vi "SubMatrixVgtmp.vi"(0 "Target Voltage, V":dbl=1.0 min=-4.0 max=4.0 step=0.1 format="%.4f", 2 "Sweep rate, V/min":dbl=0.1 min=0.0 max=1.0 step=0.01 format="%.4f", 3 "Custom Folder":string, 5 "optional Bias (V)":dbl=1e-08) -> ()   [LabVIEW 2014]
uses:
  <vilib>/Utility/file.llb/Write To Spreadsheet File (DBL).vi
panel:
  out "Comments":string[](array[string])
  out "ArrayBoolian":bool[][](array[boolean])
  out "Numeric 4":i32
  in  "Commutator":bool
  in  "Commute SorceMeter":enum32{"Radio Selection 1", "Radio Selection 2"}(radio)
  out "Numeric 3":i32
  in  "Channel 2 (Vnano3b)":bool
  in  "Channel 1 (Vnano3)":bool
  out "Numeric":i32
  in  "Capacitance (C) and Loss (L)":bool
  in  "Magnetic Field (B)":bool
  in  "Current (Ik3)":bool
  in  "Voltage (Vk3)":bool
  in  "Current (Ik2)":bool
  in  "Voltage (Vk2)":bool
  in  "Channel 2 (Vnano2b)":bool
  in  "Channel 1 (Vnano2)":bool
  in  "Thermometer 1 (T1)":bool=TRUE
  in  "Channel 2 (Vnano1b)":bool
  in  "Channel 1 (Vnano1)":bool
  in  "Current (Ik1)":bool=TRUE
  in  "Voltage (Vk1)":bool
  out "Numeric Current":dbl
  out "Main Keithly2614B address":string="12"
  out "Delib Time delay":i32
  in  "points at each Vg":i32=1
  out "XY Graph":cluster{dbl[], dbl[]}(graph)={[1.0, 0.8, 0.6000000000000001, 0.4000000000000001, 0.20000000000000007, 5.551115123125783e-17, -0.19999999999999996, -0.39999999999999997, -0.6, -0.8, -1.0], [0.03352775, 0.056811, 0.03911575, 0.04330675, -0.02468015, 0.011641600000000002, 0.10151450000000001, 0.12386675000000001, 0.08288825000000001, -0.00186266, -0.038650000000000004]}
  in  "Time btw \npoints, sec":dbl=1.0 format="%.2f"
  out "Array 2":dbl[][](array[numeric])
  out "array for data":dbl[](array[numeric])
  out "Array":string[](array[string])
  in  "Addr 1 lock-in oop":bool
  in  "Ring":u16(ring) caption="Y-axis:" items=["Vg", "I", "R1", "R1oop", "Ik1"]
  out "String":string
  out "Data file:":path
  in  "Set compliance limit, mkA":dbl=0.05 min=0.0 max=1.0 step=0.01 format="%.3f"
  in  "error in (no error)":errorcluster
  in  "Ring 3":u16(ring)=1 items=["1 kOhm", "10 kOhm", "100 kOhm", "1 Mohm", "10 mOhm"]
  in  "Ring 2":u16(ring)=3 items=["1 kOhm", "10 kOhm", "100 kOhm", "1 Mohm", "10 mOhm"]
  in  "Fixed Current mkA":dbl=1.0
  in  "Current is:":T1(radio)
  in  "Ressitance measurements?":bool=TRUE
  in  "Addr 5 lock-in oop":bool
  in  "Addr 4 lock-in oop":bool
  in  "Addr 3 lock-in oop":bool
  in  "Addr 2 lock-in oop":bool
  in  "Addr 5 lock-in":bool
  in  "Addr 4 lock-in":bool
  in  "Addr 3 lock-in":bool=TRUE
  in  "Addr 2 lock-in":bool=TRUE
  in  "Addr 1 lock-in":bool=TRUE
  # "Keithley 2400: address 12"
  # "0"
  # "SourceMeters"
  # "Nanovoltmeters"
  # "Temperature"
  # "Main"
  # "Magnetic Field"
  # "(not recommended, too slow)"
  # "Capacitance & Loss"
  # "(not recommended, too slow)"
  # "(not recommended, too slow)"
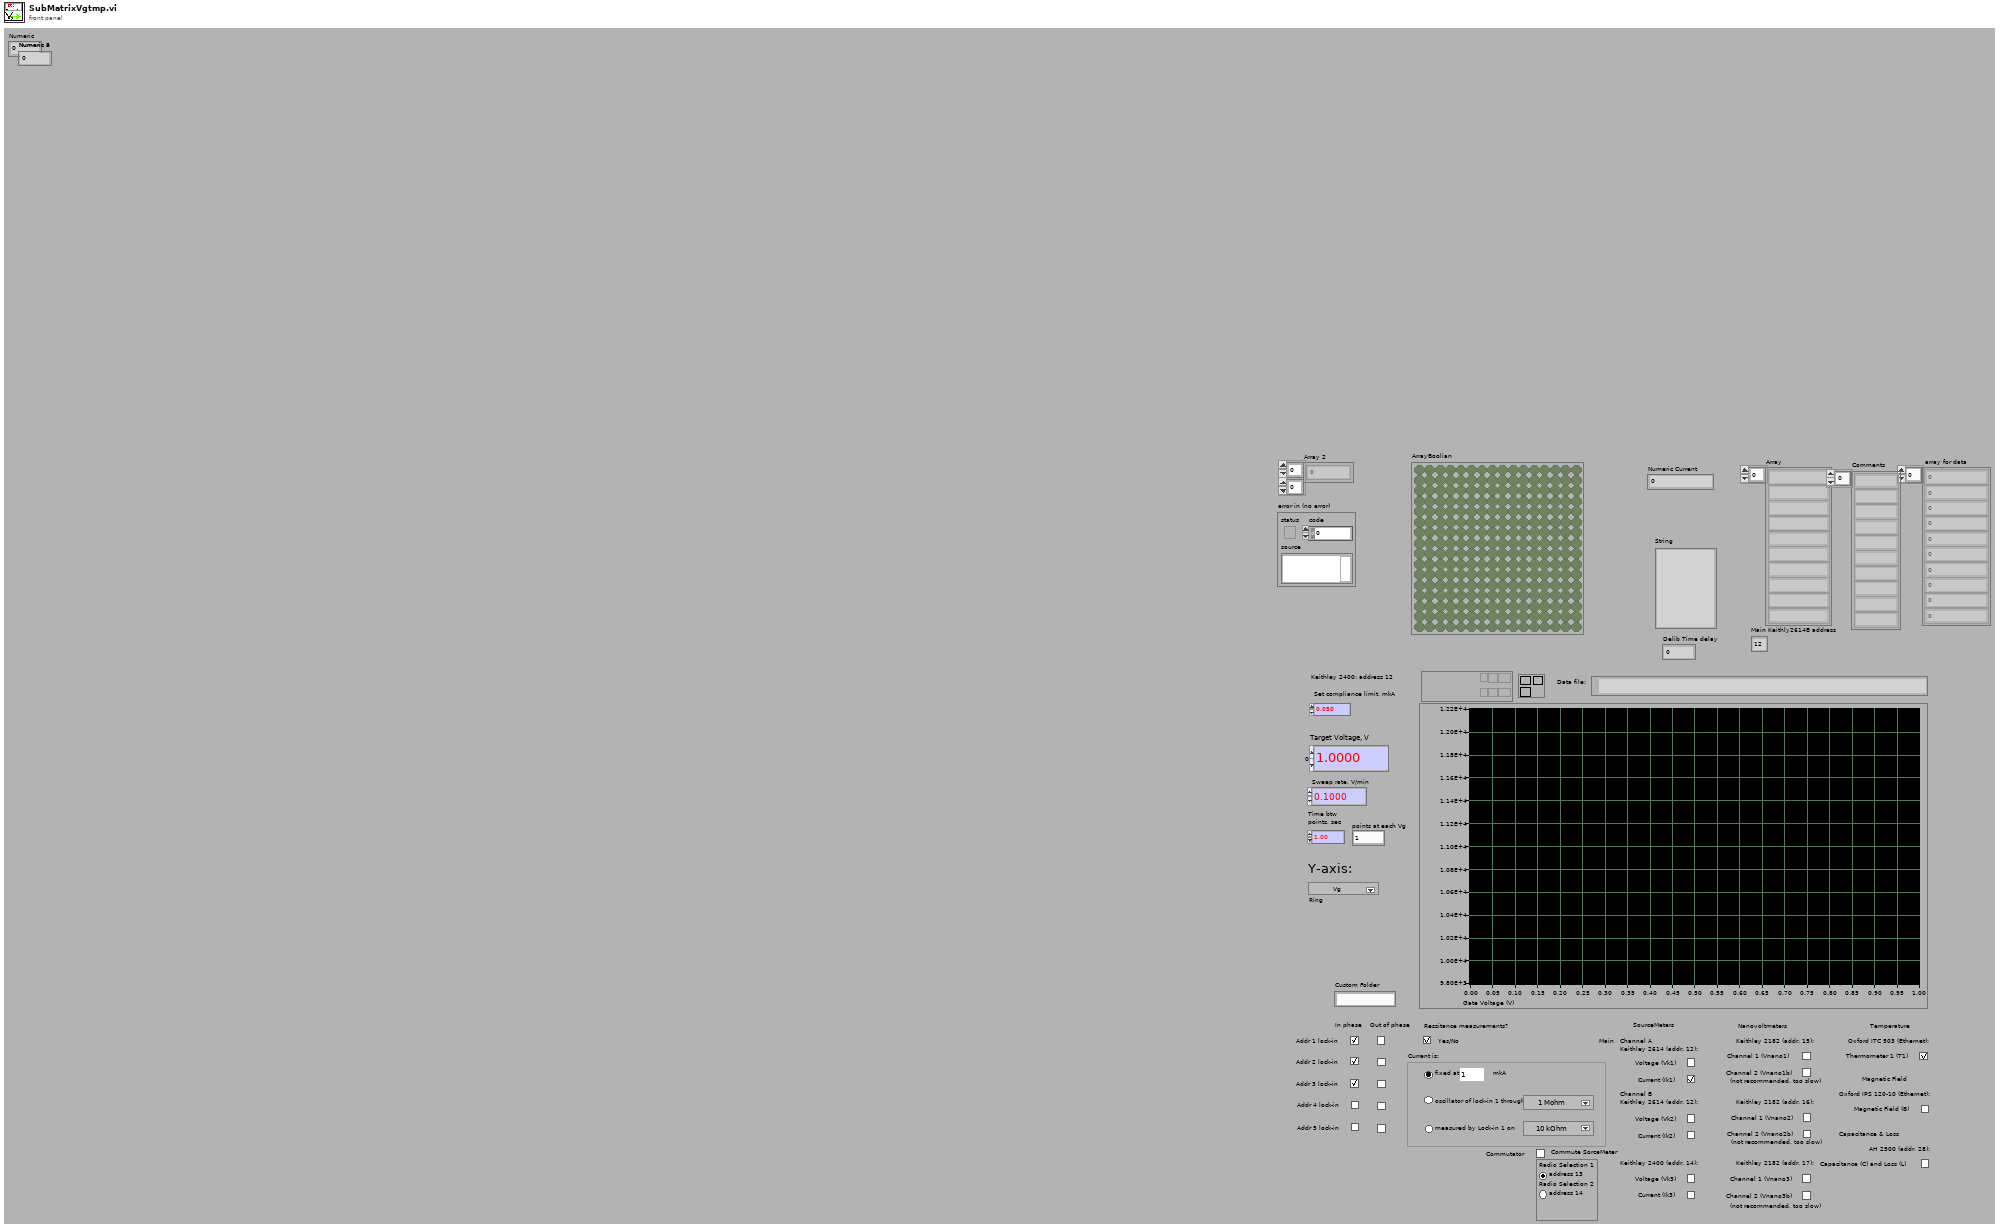
[diagram p1: front panel]
types:
  T1 = enum32{"Radio Selection 1", "Radio Selection 2", "Radio Selection 3"}
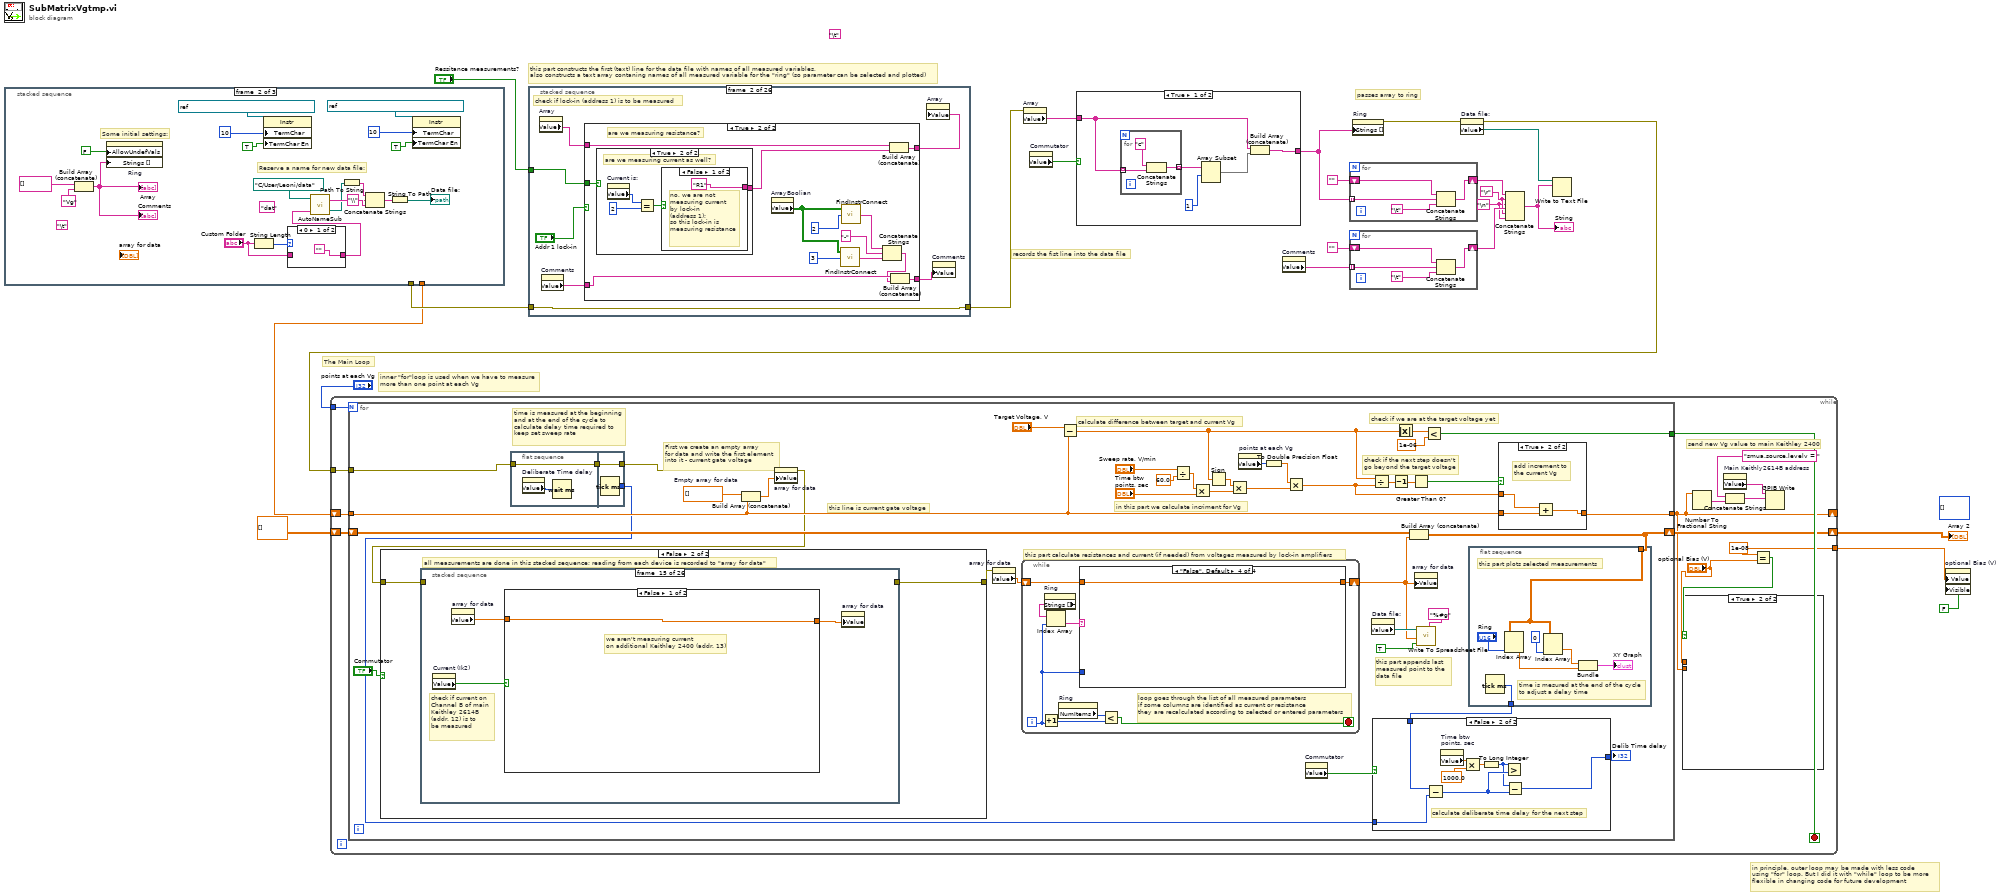
[diagram p0: block diagram]
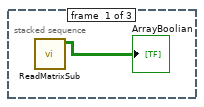
[diagram p3: hidden frame]
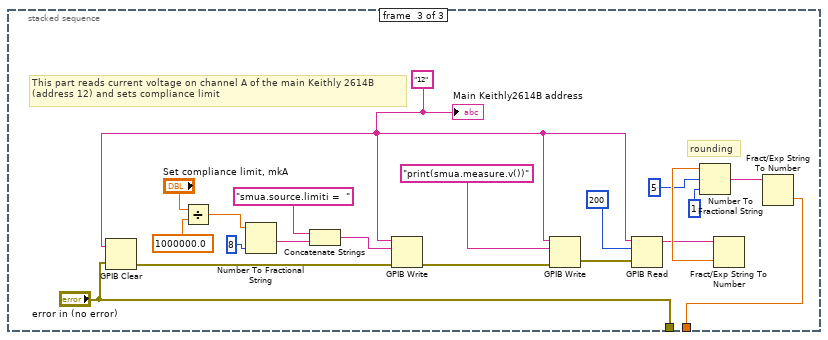
[diagram p5: hidden frame]
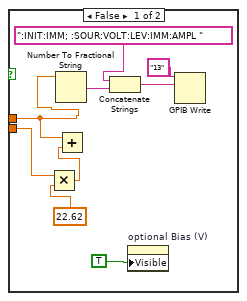
[diagram p6: hidden frame]
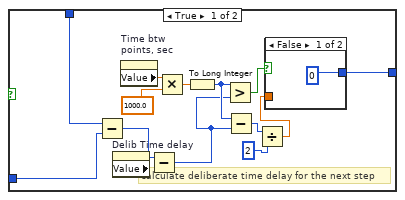
[diagram p7: hidden frame]
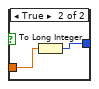
[diagram p8: hidden frame]
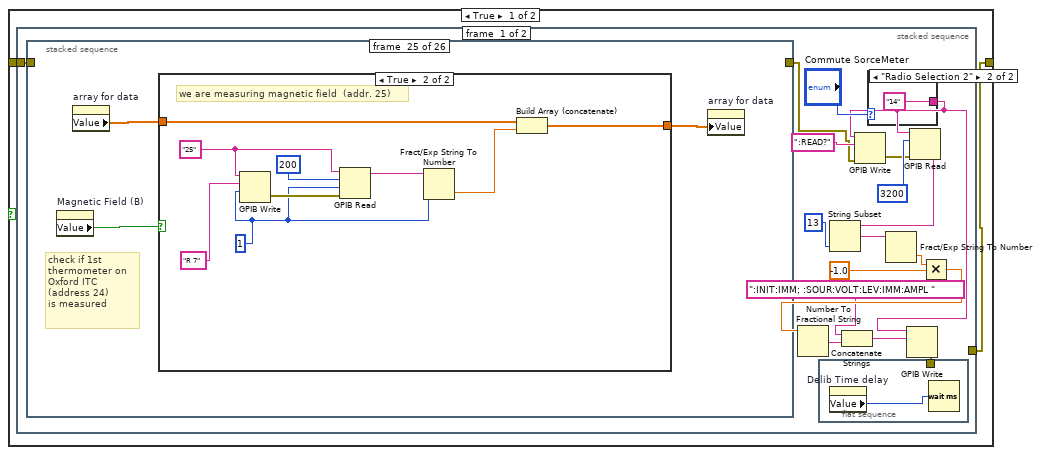
[diagram p9: hidden frame]
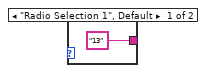
[diagram p10: hidden frame]
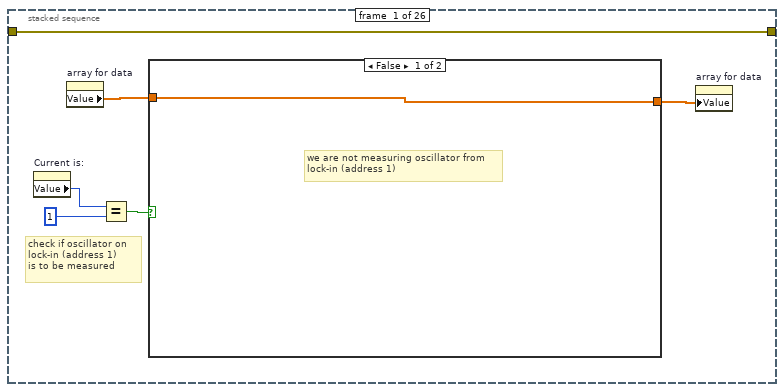
[diagram p11: hidden frame]
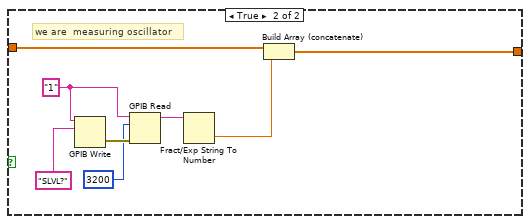
[diagram p12: hidden frame]
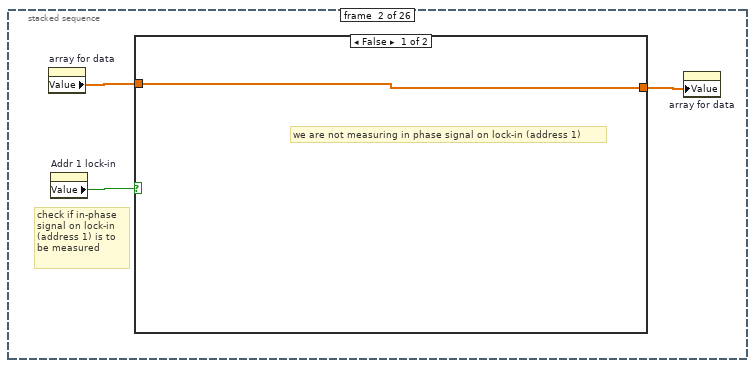
[diagram p13: hidden frame]
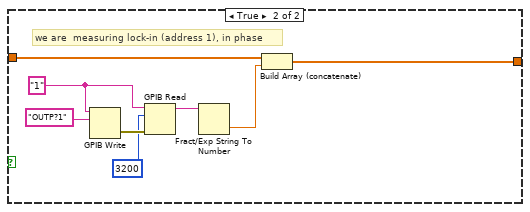
[diagram p14: hidden frame]
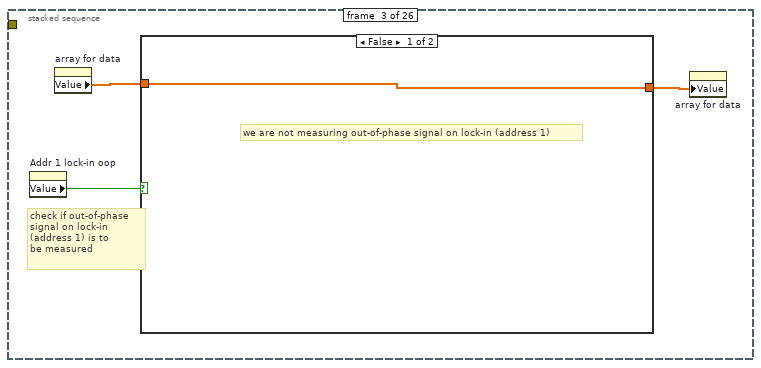
[diagram p15: hidden frame]
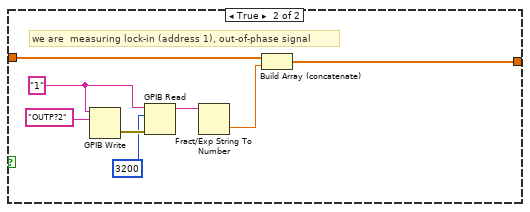
[diagram p16: hidden frame]
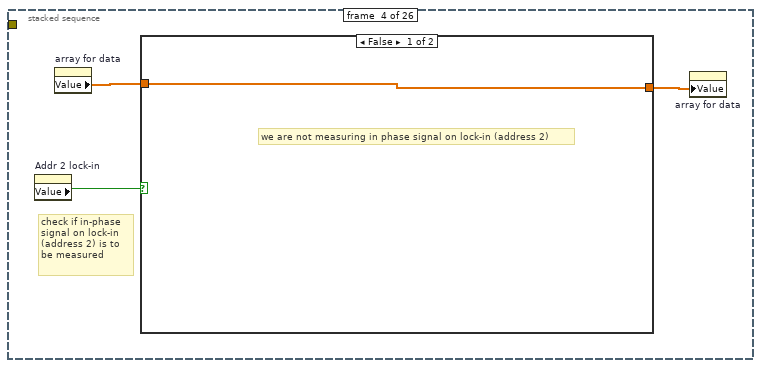
[diagram p17: hidden frame]
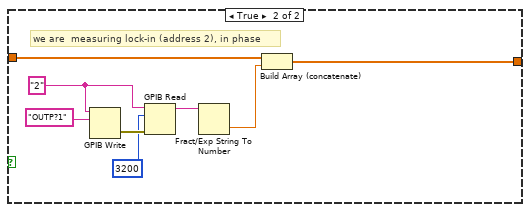
[diagram p18: hidden frame]
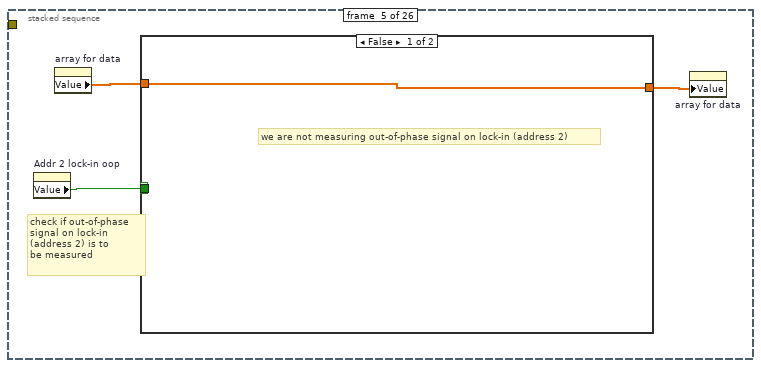
[diagram p19: hidden frame]
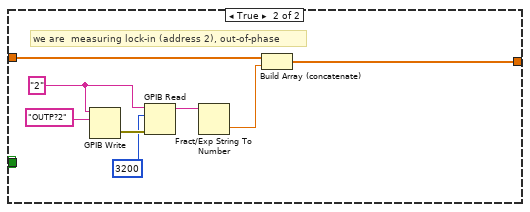
[diagram p20: hidden frame]
diagram:
  (unwired) "\t"
  w2 = "\r"
  w1 = "\n"
  (unwired) i32[][] []
  # "passes array to ring"
  # "in principle, outer loop may be made with less code\nusing \"for\" loop. But I did it with \"while\" loop to be more \nflexible in changing code for future development"
  # "inner \"for\"loop is used when we have to measure\nmore than one point at each Vg"
  # "The Main Loop"
  # "records the fist line into the data file"
  # "this part constructs the first (text) line for the data file with names of all measured variables,\nalso constructs a text array contaning names of all measured variable for the \"ring\" (so parameter can be selected and plotted)"
  n1 = stacked-sequence {
    tunnel: [_ _ "error in (no error)"] -> w23
    tunnel: [_ _ w47] -> w12
    frame #0 {
      n2 = call "ReadMatrixSub.vi"() -> ("Array"=→"ArrayBoolian":bool[][])  [unwired: 9 in, 2 out]
    }
    frame #1 {
      (unwired) "dat"
      (unwired) "\t"
      # "Some initial settings:"
      # "Reserve a name for new data file:"
      n3 = Build Array (concatenate)(string[] [], "Vg") -> (w25:string[])
      "Array" <- w25
      "Comments" <- w25
      n4 = property on="Ring" class="Ring (strict)"("AllowUndefVals"=FALSE, "Strings []"=w25) -> ()  [unwired: 2 in, 2 out]
      n5 = String Length(string="Custom Folder") -> (length=w35:i32)
      n6 = property class="Instr"(reference=refnum<visa-resource-name> "TCPIP0::192.168.128.3::7020::SOCKET" ("VISA resource name"), "TermChar"=10, "TermChar En"=TRUE) -> ()  [unwired: 1 in, 2 out]
      n7 = case shown="0" w35 {
        tunnel: "Custom Folder" -> [_ w46]
        tunnel: ["" w46] -> w33
        frame 0 {
        }
        frame 1, Default {
        }
      }
      n8 = call "AutoNameSub.vi"("Custom Folder"=w33, "User Data Folder"=path "C:/User/Leoni/data") -> ("created path"=w43:path, "String"=w44:string)  [unwired: 1 in]
      n9 = Path To String(path=w43) -> (string=w38:string)
      n10 = Concatenate Strings(w38, "\\", w44) -> (w40:string)
      n11 = String To Path(string=w40) -> (path=→"Data file:":path)
      n12 = property class="Instr"(reference=refnum<visa-resource-name> "TCPIP0::192.168.128.2::7020::SOCKET" ("VISA resource name"), "TermChar"=10, "TermChar En"=TRUE) -> ()  [unwired: 1 in, 2 out]
    }
    frame #2 {
      w54 = "12"
      # "rounding"
      # "This part reads current voltage on channel A of the main Keithly 2614B \n(address 12) and sets compliance limit"
      n13 = GPIB Clear(2:"error in (no error)", 3:w54) -> (0:w59:errorcluster)  [unwired: 1 out]
      n14 = Divide(x="Set compliance limit, mkA", y=1000000.0) -> (x/y=w65:dbl)
      n15 = Number To Fractional String(number=w65, precision (6)=i16 8) -> (F-format string=w61:string)  [unwired: 2 in]
      n16 = Concatenate Strings("smua.source.limiti =  " ("data"), w61) -> (w60:string)
      n17 = GPIB Write(0:w54, 1:w60, 3:w59) -> (6:w55:errorcluster)  [unwired: 2 in, 1 out]
      n18 = GPIB Write(0:w54, 1:"print(smua.measure.v())" ("data"), 3:w55) -> (6:w58:errorcluster)  [unwired: 2 in, 1 out]
      n19 = GPIB Read(0:w54, 1:200 ("byte count"), 3:w58) -> (5:w48:string)  [unwired: 2 in, 2 out]
      n20 = Fract/Exp String To Number(string=w48) -> (number=w52:dbl)  [unwired: 3 in, 1 out]
      n21 = Number To Fractional String(number=w52, width (-)=5, precision (6)=1) -> (F-format string=w49:string)  [unwired: 1 in]
      n22 = Fract/Exp String To Number(string=w49) -> (number=w47:dbl)  [unwired: 3 in, 1 out]
      "Main Keithly2614B address" <- w54
    }
  }
  n23 = stacked-sequence {
    tunnel: "Ressitance measurements?" -> [w74 w95 w122 w139 w159 w171 w183 w195 w207 w219 w231 _ _ _ _ _ _ _ _ _ _ _ _ _ _ _]
    tunnel: w23 -> [_ w94 _ _ _ _ _ _ _ _ _ _ _ _ _ _ _ _ _ _ _ _ _ _ _ _]
    tunnel: [_ w94 _ _ _ _ _ _ _ _ _ _ _ _ _ _ _ _ _ _ _ _ _ _ _ _] -> w20
    frame #0 {
      # "check if oscillator of  lock-in (address 1) is to be measured"
      n24 = property on="Array" class="Arr (strict)"() -> ("Value"=w70:string[])  [unwired: 2 in, 2 out]
      n25 = property on="Comments" class="Arr (strict)"() -> ("Value"=w67:string[])  [unwired: 2 in, 2 out]
      n26 = Equal?(x="Current is:", y=1) -> (x = y?=w72:bool)
      n27 = case shown="True" w72 {
        tunnel: w74 -> [_ _]
        tunnel: w70 -> [w76 w87]
        tunnel: [w76 w86] -> w69
        tunnel: [w75 w79] -> w68
        tunnel: w67 -> [w75 w78]
        frame False {
          # "we are not measuring oscillator from\nlock-in (address 1)"
        }
        frame True {
          # "This subVI takes the matrix column # (instrument\nconnection point) as an argument and finds the raw\n# (contact) to which the instrument is connected"
          # "we are  measuring oscillator"
          n28 = property on="ArrayBoolian" class="Arr (strict)"() -> ("Value"=w83:bool[][])  [unwired: 2 in, 2 out]
          n29 = GPIB Clear(3:"1") -> ()  [unwired: 1 in, 2 out]
          n30 = call "FindInstrConnect.vi"("Column #"=1, "ArrayBoolian"=w83) -> ("String"=w84:string)  [unwired: 1 in, 2 out]
          n31 = call "FindInstrConnect.vi"("Column #"=0, "ArrayBoolian"=w83) -> ("String"=w81:string)  [unwired: 1 in, 2 out]
          n32 = Concatenate Strings(w81, "-", w84) -> (w77:string)
          n33 = Build Array (concatenate)(w87, "I") -> (w86:string[])
          n34 = Build Array (concatenate)(w78, w77) -> (w79:string[])
        }
      }
      n35 = property on="Comments" class="Arr (strict)"("Value"=w68) -> ()  [unwired: 2 in, 2 out]
      n36 = property on="Array" class="Arr (strict)"("Value"=w69) -> ()  [unwired: 2 in, 2 out]
    }
    frame #1 {
      # "check if lock-in (address 1) is to be measured"
      n37 = property on="Array" class="Arr (strict)"() -> ("Value"=w93:string[])  [unwired: 2 in, 2 out]
      n38 = property on="Comments" class="Arr (strict)"() -> ("Value"=w91:string[])  [unwired: 2 in, 2 out]
      n39 = case shown="True" "Addr 1 lock-in" {
        tunnel: w95 -> [_ w111]
        tunnel: w93 -> [w98 w109]
        tunnel: [w98 w110] -> w92
        tunnel: w91 -> [w97 w100]
        tunnel: [w97 w101] -> w90
        frame False {
          # "we are not measuring in phase signal from\nlock-in (address 1)"
        }
        frame True {
          # "are we measuring resistance?"
          n40 = case shown="True" w111 {
            tunnel: ["V1" w113] -> w102
            frame False {
              # "no, we are not measuring resistanse;\nall lock-ins are measuring voltage"
            }
            frame True {
              # "are we measuring current as well?"
              n41 = property on="Current is:" class="RadioBtnsControl (strict)"() -> ("Value"=w115:T1)  [unwired: 2 in, 2 out]
              n42 = Equal?(x=w115, y=2) -> (x = y?=w116:bool)
              n43 = case shown="False" w116 {
                tunnel: ["R1" "I"] -> w113
                frame False {
                  # "no, we are not \nmeasuring current\nby lock-in \n(address 1); \nso this lock-in is \nmeasuring resistance"
                }
                frame True {
                  # "yes, we are measuring \ncurrent by lock-in \n(address 1) as \nvoltage drop on \nknown resistance"
                }
              }
            }
          }
          n44 = property on="ArrayBoolian" class="Arr (strict)"() -> ("Value"=w103:bool[][])  [unwired: 2 in, 2 out]
          n45 = call "FindInstrConnect.vi"("Column #"=3, "ArrayBoolian"=w103) -> ("String"=w106:string)  [unwired: 1 in, 2 out]
          n46 = call "FindInstrConnect.vi"("Column #"=2, "ArrayBoolian"=w103) -> ("String"=w104:string)  [unwired: 1 in, 2 out]
          n47 = Concatenate Strings(w104, "-", w106) -> (w99:string)
          n48 = Build Array (concatenate)(w109, w102) -> (w110:string[])
          n49 = Build Array (concatenate)(w100, w99) -> (w101:string[])
        }
      }
      n50 = property on="Array" class="Arr (strict)"("Value"=w92) -> ()  [unwired: 2 in, 2 out]
      n51 = property on="Comments" class="Arr (strict)"("Value"=w90) -> ()  [unwired: 2 in, 2 out]
    }
    frame #2 {
      # "check if out-of-phase signal on  lock-in (address 1) is to be measured"
      n52 = property on="Array" class="Arr (strict)"() -> ("Value"=w121:string[])  [unwired: 2 in, 2 out]
      n53 = case shown="True" "Addr 1 lock-in oop" {
        tunnel: w122 -> [_ w128]
        tunnel: w121 -> [w123 w125]
        tunnel: [w123 w126] -> w120
        frame False {
          # "we are not measuring iout-of-phase signal from\nlock-in (address 1)"
        }
        frame True {
          # "are we measuring resistance?"
          n54 = GPIB Clear(3:"1") -> ()  [unwired: 1 in, 2 out]
          n55 = case shown="True" w128 {
            tunnel: ["V1oop" w130] -> w124
            frame False {
              # "no, we are not measuring resistance;\nall lock-ins are measuring voltage"
            }
            frame True {
              # "are we measuring out-of-phase current as well?"
              n56 = property on="Current is:" class="RadioBtnsControl (strict)"() -> ("Value"=w132:T1)  [unwired: 2 in, 2 out]
              n57 = Equal?(x=w132, y=2) -> (x = y?=w133:bool)
              n58 = case shown="False" w133 {
                tunnel: ["R1oop" "Ioop"] -> w130
                frame False {
                  # "no, we are not \nmeasuring current\nby lock-in \n(address 1); so this \nlock-in is measuring\nout-of-phase resistance"
                }
                frame True {
                  # "yes, we are measuring \nout-of phase current \nby lock-in (address 1) \nas voltage drop on \nknown resistance"
                }
              }
            }
          }
          n59 = Build Array (concatenate)(w125, w124) -> (w126:string[])
        }
      }
      n60 = property on="Array" class="Arr (strict)"("Value"=w120) -> ()  [unwired: 2 in, 2 out]
    }
    frame #3 {
      # "check if in-phase signal on  lock-in (address 2) is to be measured"
      n61 = property on="Array" class="Arr (strict)"() -> ("Value"=w138:string[])  [unwired: 2 in, 2 out]
      n62 = case shown="True" "Addr 2 lock-in" {
        tunnel: w139 -> [_ w153]
        tunnel: w138 -> [w140 w150]
        tunnel: [w140 w151] -> w137
        frame False {
          # "we are not measuring in-phase signal from\nlock-in (address 2)"
        }
        frame True {
          (unwired) "\t"
          # "are we measuring resistance?"
          n63 = GPIB Clear(3:"2") -> ()  [unwired: 1 in, 2 out]
          n64 = case shown="False" w153 {
            tunnel: ["R2 (" "V2 ("] -> w142
            frame True {
              # "we are measuring \nresistance by lock-in \n(address 2)"
            }
            frame False, Default {
              # "no, we are not \nmeasuring resistance;\nall lock-ins are \nmeasuring voltage"
            }
          }
          n65 = property on="ArrayBoolian" class="Arr (strict)"() -> ("Value"=w141:bool[][])  [unwired: 2 in, 2 out]
          n66 = call "FindInstrConnect.vi"("Column #"=5, "ArrayBoolian"=w141) -> ("String"=w146:string)  [unwired: 1 in, 2 out]
          n67 = call "FindInstrConnect.vi"("Column #"=4, "ArrayBoolian"=w141) -> ("String"=w144:string)  [unwired: 1 in, 2 out]
          n68 = Concatenate Strings(w142, w144, "-", w146, ")") -> (w143:string)
          n69 = Build Array (concatenate)(w150, w143) -> (w151:string[])
        }
      }
      n70 = property on="Array" class="Arr (strict)"("Value"=w137) -> ()  [unwired: 2 in, 2 out]
    }
    frame #4 {
      # "check if out-of-phase signal on  lock-in (address 2) is to be measured"
      n71 = property on="Array" class="Arr (strict)"() -> ("Value"=w158:string[])  [unwired: 2 in, 2 out]
      n72 = case shown="False" "Addr 2 lock-in oop" {
        tunnel: w159 -> [_ w165]
        tunnel: w158 -> [w160 w162]
        tunnel: [w160 w163] -> w157
        frame False {
          # "we are not measuring out-of-phase signal from\nlock-in (address 2)"
        }
        frame True {
          (unwired) "\t"
          # "are we measuring resistance?"
          n73 = GPIB Clear(3:"2") -> ()  [unwired: 1 in, 2 out]
          n74 = case shown="True" w165 {
            tunnel: ["R2oop" "V2oop"] -> w161
            frame True {
              # "we are measuring out-of-phase resistance by lock-in (address 2)\n(address 2)"
            }
            frame False, Default {
              # "no, we are not measuring resistance;\nall lock-ins are measuring voltage"
            }
          }
          n75 = Build Array (concatenate)(w162, w161) -> (w163:string[])
        }
      }
      n76 = property on="Array" class="Arr (strict)"("Value"=w157) -> ()  [unwired: 2 in, 2 out]
    }
    frame #5 {
      # "check if in-phase signal on  lock-in (address 3) is to be measured"
      n77 = property on="Array" class="Arr (strict)"() -> ("Value"=w170:string[])  [unwired: 2 in, 2 out]
      n78 = case shown="True" "Addr 3 lock-in" {
        tunnel: w171 -> [_ w177]
        tunnel: w170 -> [w172 w174]
        tunnel: [w172 w175] -> w169
        frame False {
          # "we are not measuring in-phase signal from\nlock-in (address 3)"
        }
        frame True {
          (unwired) "\t"
          # "are we measuring resistance?"
          n79 = GPIB Clear(3:"3") -> ()  [unwired: 1 in, 2 out]
          n80 = case shown="True" w177 {
            tunnel: ["R3" "V3"] -> w173
            frame True {
              # "we are measuring \nresistance by lock-in \n(address 3)"
            }
            frame False, Default {
              # "no, we are not measuring resistance;\nall lock-ins are measuring voltage"
            }
          }
          n81 = Build Array (concatenate)(w174, w173) -> (w175:string[])
        }
      }
      n82 = property on="Array" class="Arr (strict)"("Value"=w169) -> ()  [unwired: 2 in, 2 out]
    }
    frame #6 {
      # "check if out-of-phase signal on  lock-in (address 3) is to be measured"
      n83 = property on="Array" class="Arr (strict)"() -> ("Value"=w182:string[])  [unwired: 2 in, 2 out]
      n84 = case shown="False" "Addr 3 lock-in oop" {
        tunnel: w183 -> [_ w189]
        tunnel: w182 -> [w184 w186]
        tunnel: [w184 w187] -> w181
        frame False {
          # "we are not measuring out-of-phase signal from\nlock-in (address 3)"
        }
        frame True {
          (unwired) "\t"
          # "are we measuring resistance?"
          n85 = GPIB Clear(3:"3") -> ()  [unwired: 1 in, 2 out]
          n86 = case shown="True" w189 {
            tunnel: ["R3oop" "V3oop"] -> w185
            frame True {
              # "we are measuring out-of-phase resistance by lock-in (address 3)\n(address 2)"
            }
            frame False, Default {
              # "no, we are not measuring resistance;\nall lock-ins are measuring voltage"
            }
          }
          n87 = Build Array (concatenate)(w186, w185) -> (w187:string[])
        }
      }
      n88 = property on="Array" class="Arr (strict)"("Value"=w181) -> ()  [unwired: 2 in, 2 out]
    }
    frame #7 {
      # "check if in-phase signal on  lock-in (address 4) is to be measured"
      n89 = property on="Array" class="Arr (strict)"() -> ("Value"=w194:string[])  [unwired: 2 in, 2 out]
      n90 = case shown="False" "Addr 4 lock-in" {
        tunnel: w195 -> [_ w201]
        tunnel: w194 -> [w196 w198]
        tunnel: [w196 w199] -> w193
        frame False {
          # "we are not measuring in-phase signal from\nlock-in (address 4)"
        }
        frame True {
          (unwired) "\t"
          # "are we measuring resistance?"
          n91 = GPIB Clear(3:"4") -> ()  [unwired: 1 in, 2 out]
          n92 = case shown="True" w201 {
            tunnel: ["R4" "V4"] -> w197
            frame True {
              # "we are measuring \nresistance by lock-in \n(address 4)"
            }
            frame False, Default {
              # "no, we are not measuring resistance;\nall lock-ins are measuring voltage"
            }
          }
          n93 = Build Array (concatenate)(w198, w197) -> (w199:string[])
        }
      }
      n94 = property on="Array" class="Arr (strict)"("Value"=w193) -> ()  [unwired: 2 in, 2 out]
    }
    frame #8 {
      # "check if out-of-phase signal on  lock-in (address 4) is to be measured"
      n95 = property on="Array" class="Arr (strict)"() -> ("Value"=w206:string[])  [unwired: 2 in, 2 out]
      n96 = case shown="False" "Addr 4 lock-in oop" {
        tunnel: w207 -> [_ w213]
        tunnel: w206 -> [w208 w210]
        tunnel: [w208 w211] -> w205
        frame False {
          # "we are not measuring out-of-phase signal from\nlock-in (address 4)"
        }
        frame True {
          (unwired) "\t"
          # "are we measuring resistance?"
          n97 = GPIB Clear(3:"4") -> ()  [unwired: 1 in, 2 out]
          n98 = case shown="True" w213 {
            tunnel: ["R4oop" "V4oop"] -> w209
            frame True {
              # "we are measuring out-of-phase resistance by lock-in (address 4)\n(address 2)"
            }
            frame False, Default {
              # "no, we are not measuring resistance;\nall lock-ins are measuring voltage"
            }
          }
          n99 = Build Array (concatenate)(w210, w209) -> (w211:string[])
        }
      }
      n100 = property on="Array" class="Arr (strict)"("Value"=w205) -> ()  [unwired: 2 in, 2 out]
    }
    frame #9 {
      # "check if in-phase signal on  lock-in (address 5) is to be measured"
      n101 = property on="Array" class="Arr (strict)"() -> ("Value"=w218:string[])  [unwired: 2 in, 2 out]
      n102 = case shown="False" "Addr 5 lock-in" {
        tunnel: w219 -> [_ w225]
        tunnel: w218 -> [w220 w222]
        tunnel: [w220 w223] -> w217
        frame False {
          # "we are not measuring in-phase signal from\nlock-in (address 5)"
        }
        frame True {
          (unwired) "\t"
          # "are we measuring resistance?"
          n103 = GPIB Clear(3:"5") -> ()  [unwired: 1 in, 2 out]
          n104 = case shown="True" w225 {
            tunnel: ["R5" "V5"] -> w221
            frame True {
              # "we are measuring \nresistance by lock-in \n(address 5)"
            }
            frame False, Default {
              # "no, we are not measuring resistance;\nall lock-ins are measuring voltage"
            }
          }
          n105 = Build Array (concatenate)(w222, w221) -> (w223:string[])
        }
      }
      n106 = property on="Array" class="Arr (strict)"("Value"=w217) -> ()  [unwired: 2 in, 2 out]
    }
    frame #10 {
      # "check if out-of-phase signal on  lock-in (address 5) is to be measured"
      n107 = property on="Array" class="Arr (strict)"() -> ("Value"=w230:string[])  [unwired: 2 in, 2 out]
      n108 = case shown="True" "Addr 5 lock-in oop" {
        tunnel: w231 -> [_ w237]
        tunnel: w230 -> [w232 w234]
        tunnel: [w232 w235] -> w229
        frame False {
          # "we are not measuring out-of-phase signal from\nlock-in (address 5)"
        }
        frame True {
          (unwired) "\t"
          # "are we measuring resistance?"
          n109 = GPIB Clear(3:"5") -> ()  [unwired: 1 in, 2 out]
          n110 = case shown="True" w237 {
            tunnel: ["R5oop" "V5oop"] -> w233
            frame True {
              # "we are measuring out-of-phase resistance by lock-in (address 5)\n(address 2)"
            }
            frame False, Default {
              # "no, we are not measuring resistance;\nall lock-ins are measuring voltage"
            }
          }
          n111 = Build Array (concatenate)(w234, w233) -> (w235:string[])
        }
      }
      n112 = property on="Array" class="Arr (strict)"("Value"=w229) -> ()  [unwired: 2 in, 2 out]
    }
    frame #11 {
      # "check if voltage on main Keithley 2400 (addr. 12) is measured"
      n113 = property on="Array" class="Arr (strict)"() -> ("Value"=w242:string[])  [unwired: 2 in, 2 out]
      n114 = case shown="False" "Voltage (Vk1)" {
        tunnel: w242 -> [w243 w245]
        tunnel: [w243 w246] -> w241
        frame False {
          # "no , we aren't measuring voltage \non main Keithley 2400 (addr. 12)"
        }
        frame True {
          (unwired) "\t"
          # "yes , we are measuring voltage \non main Keithley 2400 (addr. 12)"
          n115 = GPIB Clear(3:"12") -> ()  [unwired: 1 in, 2 out]
          n116 = Build Array (concatenate)(w245, "Vk1") -> (w246:string[])
        }
      }
      n117 = property on="Array" class="Arr (strict)"("Value"=w241) -> ()  [unwired: 2 in, 2 out]
    }
    frame #12 {
      # "check if current on main Keithley 2400 (addr. 12) is measured"
      n118 = property on="Array" class="Arr (strict)"() -> ("Value"=w250:string[])  [unwired: 2 in, 2 out]
      n119 = case shown="True" "Current (Ik1)" {
        tunnel: w250 -> [w251 w253]
        tunnel: [w251 w254] -> w249
        frame False {
          # "no , we aren't measuring current\non main Keithley 2400 (addr. 12)"
        }
        frame True {
          (unwired) "\t"
          # "yes , we are measuring current \non main Keithley 2400 (addr. 12)"
          n120 = GPIB Clear(3:"12") -> ()  [unwired: 1 in, 2 out]
          n121 = Build Array (concatenate)(w253, "Ik1") -> (w254:string[])
        }
      }
      n122 = property on="Array" class="Arr (strict)"("Value"=w249) -> ()  [unwired: 2 in, 2 out]
    }
    frame #13 {
      # "check if voltage on additional Keithley 2400 (addr. 13) is measured"
      n123 = property on="Array" class="Arr (strict)"() -> ("Value"=w258:string[])  [unwired: 2 in, 2 out]
      n124 = case shown="False" "Voltage (Vk2)" {
        tunnel: w258 -> [w259 w261]
        tunnel: [w259 w262] -> w257
        frame False {
          # "no , we aren't measuring voltage \non Keithley 2400 (addr. 13)"
        }
        frame True {
          (unwired) "\t"
          # "yes , we are measuring voltage \non Keithley 2400 (addr. 13)"
          n125 = GPIB Clear(3:"13") -> ()  [unwired: 1 in, 2 out]
          n126 = Build Array (concatenate)(w261, "Vk2") -> (w262:string[])
        }
      }
      n127 = property on="Array" class="Arr (strict)"("Value"=w257) -> ()  [unwired: 2 in, 2 out]
    }
    frame #14 {
      # "check if current on additional Keithley 2400 (addr. 13) is measured"
      n128 = property on="Array" class="Arr (strict)"() -> ("Value"=w266:string[])  [unwired: 2 in, 2 out]
      n129 = case shown="False" "Current (Ik2)" {
        tunnel: w266 -> [w267 w269]
        tunnel: [w267 w270] -> w265
        frame False {
          # "no , we aren't measuring current\non Keithley 2400 (addr. 13)"
        }
        frame True {
          (unwired) "\t"
          # "yes , we are measuring current \non Keithley 2400 (addr. 13)"
          n130 = GPIB Clear(3:"13") -> ()  [unwired: 1 in, 2 out]
          n131 = Build Array (concatenate)(w269, "Ik2") -> (w270:string[])
        }
      }
      n132 = property on="Array" class="Arr (strict)"("Value"=w265) -> ()  [unwired: 2 in, 2 out]
    }
    frame #15 {
      # "check if voltage on additional Keithley 2400 (addr. 14) is measured"
      n133 = property on="Array" class="Arr (strict)"() -> ("Value"=w274:string[])  [unwired: 2 in, 2 out]
      n134 = case shown="False" "Voltage (Vk3)" {
        tunnel: w274 -> [w275 w277]
        tunnel: [w275 w278] -> w273
        frame False {
          # "no , we aren't measuring voltage \non Keithley 2400 (addr. 14)"
        }
        frame True {
          (unwired) "\t"
          # "yes , we are measuring voltage \non Keithley 2400 (addr. 14)"
          n135 = GPIB Clear(3:"14") -> ()  [unwired: 1 in, 2 out]
          n136 = Build Array (concatenate)(w277, "Vk3") -> (w278:string[])
        }
      }
      n137 = property on="Array" class="Arr (strict)"("Value"=w273) -> ()  [unwired: 2 in, 2 out]
    }
    frame #16 {
      # "check if current on additional Keithley 2400 (addr. 14) is measured"
      n138 = property on="Array" class="Arr (strict)"() -> ("Value"=w282:string[])  [unwired: 2 in, 2 out]
      n139 = case shown="False" "Current (Ik3)" {
        tunnel: w282 -> [w283 w285]
        tunnel: [w283 w286] -> w281
        frame False {
          # "no , we aren't measuring current\non Keithley 2400 (addr. 14)"
        }
        frame True {
          (unwired) "\t"
          # "yes , we are measuring current \non Keithley 2400 (addr. 14)"
          n140 = GPIB Clear(3:"14") -> ()  [unwired: 1 in, 2 out]
          n141 = Build Array (concatenate)(w285, "Ik3") -> (w286:string[])
        }
      }
      n142 = property on="Array" class="Arr (strict)"("Value"=w281) -> ()  [unwired: 2 in, 2 out]
    }
    frame #17 {
      # "check if 1st channel of nanovoltmeter Keithley 2182 (addr. 15) is measured"
      n143 = property on="Array" class="Arr (strict)"() -> ("Value"=w290:string[])  [unwired: 2 in, 2 out]
      n144 = case shown="False" "Channel 1 (Vnano1)" {
        tunnel: w290 -> [w291 w294]
        tunnel: [w291 w295] -> w289
        frame False {
          # "no , we are not measuring 1st channel\non Keithley 2182 (addr. 15)"
        }
        frame True {
          (unwired) "\t"
          # "yes , we are measuring 1st channel\non Keithley 2182 (addr. 15)"
          n145 = GPIB Clear(3:"15") -> ()  [unwired: 1 in, 2 out]
          n146 = Build Array (concatenate)(w294, "Vnano1") -> (w295:string[])
        }
      }
      n147 = property on="Array" class="Arr (strict)"("Value"=w289) -> ()  [unwired: 2 in, 2 out]
    }
    frame #18 {
      # "check if 2nd channel of nanovoltmeter Keithley 2182 (addr. 15) is measured"
      n148 = property on="Array" class="Arr (strict)"() -> ("Value"=w298:string[])  [unwired: 2 in, 2 out]
      n149 = case shown="False" "Channel 2 (Vnano1b)" {
        tunnel: w298 -> [w299 w301]
        tunnel: [w299 w302] -> w297
        frame False {
          # "no , we are not measuring 2nd channel\non Keithley 2182 (addr. 15)"
        }
        frame True {
          (unwired) "\t"
          # "yes , we are measuring 2nd channel\non Keithley 2182 (addr. 15)"
          n150 = GPIB Clear(3:"15") -> ()  [unwired: 1 in, 2 out]
          n151 = Build Array (concatenate)(w301, "Vnano1b") -> (w302:string[])
        }
      }
      n152 = property on="Array" class="Arr (strict)"("Value"=w297) -> ()  [unwired: 2 in, 2 out]
    }
    frame #19 {
      # "check if 1st channel of nanovoltmeter Keithley 2182 (addr. 16) is measured"
      n153 = property on="Array" class="Arr (strict)"() -> ("Value"=w306:string[])  [unwired: 2 in, 2 out]
      n154 = case shown="False" "Channel 1 (Vnano2)" {
        tunnel: w306 -> [w307 w310]
        tunnel: [w307 w311] -> w305
        frame False {
          # "no , we are not measuring 1st channel\non Keithley 2182 (addr. 16)"
        }
        frame True {
          (unwired) "\t"
          # "yes , we are measuring 1st channel\non Keithley 2182 (addr. 16)"
          n155 = GPIB Clear(3:"16") -> ()  [unwired: 1 in, 2 out]
          n156 = Build Array (concatenate)(w310, "Vnano2") -> (w311:string[])
        }
      }
      n157 = property on="Array" class="Arr (strict)"("Value"=w305) -> ()  [unwired: 2 in, 2 out]
    }
    frame #20 {
      # "check if 2nd channel of nanovoltmeter Keithley 2182 (addr. 16) is measured"
      n158 = property on="Array" class="Arr (strict)"() -> ("Value"=w314:string[])  [unwired: 2 in, 2 out]
      n159 = case shown="False" "Channel 2 (Vnano2b)" {
        tunnel: w314 -> [w315 w317]
        tunnel: [w315 w318] -> w313
        frame False {
          # "no , we are not measuring 2nd channel\non Keithley 2182 (addr. 16)"
        }
        frame True {
          (unwired) "\t"
          # "yes , we are measuring 2nd channel\non Keithley 2182 (addr. 16)"
          n160 = GPIB Clear(3:"16") -> ()  [unwired: 1 in, 2 out]
          n161 = Build Array (concatenate)(w317, "Vnano2b") -> (w318:string[])
        }
      }
      n162 = property on="Array" class="Arr (strict)"("Value"=w313) -> ()  [unwired: 2 in, 2 out]
    }
    frame #21 {
      # "check if 1st channel of nanovoltmeter Keithley 2182 (addr. 17) is measured"
      n163 = property on="Array" class="Arr (strict)"() -> ("Value"=w322:string[])  [unwired: 2 in, 2 out]
      n164 = case shown="False" "Channel 1 (Vnano3)" {
        tunnel: w322 -> [w323 w325]
        tunnel: [w323 w326] -> w321
        frame False {
          # "no , we are not measuring 1st channel\non Keithley 2182 (addr. 17)"
        }
        frame True {
          (unwired) "\t"
          # "yes , we are measuring 1st channel\non Keithley 2182 (addr. 17)"
          n165 = GPIB Clear(3:"17") -> ()  [unwired: 1 in, 2 out]
          n166 = Build Array (concatenate)(w325, "Vnano3") -> (w326:string[])
        }
      }
      n167 = property on="Array" class="Arr (strict)"("Value"=w321) -> ()  [unwired: 2 in, 2 out]
    }
    frame #22 {
      # "check if 2nd channel of nanovoltmeter Keithley 2182 (addr. 16) is measured"
      n168 = property on="Array" class="Arr (strict)"() -> ("Value"=w330:string[])  [unwired: 2 in, 2 out]
      n169 = case shown="False" "Channel 2 (Vnano3b)" {
        tunnel: w330 -> [w331 w333]
        tunnel: [w331 w334] -> w329
        frame False {
          # "no , we are not measuring 2nd channel\non Keithley 2182 (addr. 17)"
        }
        frame True {
          (unwired) "\t"
          # "yes , we are measuring 2nd channel\non Keithley 2182 (addr. 17)"
          n170 = GPIB Clear(3:"17") -> ()  [unwired: 1 in, 2 out]
          n171 = Build Array (concatenate)(w333, "Vnano3b") -> (w334:string[])
        }
      }
      n172 = property on="Array" class="Arr (strict)"("Value"=w329) -> ()  [unwired: 2 in, 2 out]
    }
    frame #23 {
      # "check if 1st thermometer on Oxford ITC (address 24) is measured"
      n173 = property on="Array" class="Arr (strict)"() -> ("Value"=w338:string[])  [unwired: 2 in, 2 out]
      n174 = case shown="False" "Thermometer 1 (T1)" {
        tunnel: w338 -> [w339 w341]
        tunnel: [w339 w342] -> w337
        frame False {
          # "no, we are not measuring temperature\non thermometer 1 (addr. 24)"
        }
        frame True {
          (unwired) "\t"
          # "yes, we are measuring temperature,\nthermometer 1 (addr. 24)"
          n175 = GPIB Clear(3:"24") -> ()  [unwired: 1 in, 2 out]
          n176 = Build Array (concatenate)(w341, "T1") -> (w342:string[])
        }
      }
      n177 = property on="Array" class="Arr (strict)"("Value"=w337) -> ()  [unwired: 2 in, 2 out]
    }
    frame #24 {
      # "check if magnetic field from Oxford IPS 120 (address 25) is measured"
      n178 = property on="Array" class="Arr (strict)"() -> ("Value"=w346:string[])  [unwired: 2 in, 2 out]
      n179 = case shown="False" "Magnetic Field (B)" {
        tunnel: w346 -> [w347 w349]
        tunnel: [w347 w350] -> w345
        frame False {
          # "no, we are not measuring magnetic field  (addr. 25)"
        }
        frame True {
          (unwired) "\t"
          # "yes, we are measuring magnetic field  (addr. 25)"
          n180 = GPIB Clear(3:"25") -> ()  [unwired: 1 in, 2 out]
          n181 = Build Array (concatenate)(w349, "B") -> (w350:string[])
        }
      }
      n182 = property on="Array" class="Arr (strict)"("Value"=w345) -> ()  [unwired: 2 in, 2 out]
    }
    frame #25 {
      # "check if capacitance and loss from AH 2500 (address 28) are measured"
      n183 = property on="Array" class="Arr (strict)"() -> ("Value"=w354:string[])  [unwired: 2 in, 2 out]
      n184 = case shown="False" "Capacitance (C) and Loss (L)" {
        tunnel: w354 -> [w355 w357]
        tunnel: [w355 w360] -> w353
        frame False {
          # "no, we are not measuring capacitance  (addr. 28)"
        }
        frame True {
          (unwired) "\t"
          (unwired) "\t"
          # "yes, we are measuring capacitance and loss  (addr. 28)"
          n185 = GPIB Clear(3:"28") -> ()  [unwired: 1 in, 2 out]
          n186 = Build Array (concatenate)(w357, "C") -> (w356:string[])
          n187 = Build Array (concatenate)(w356, "L") -> (w360:string[])
        }
      }
      n188 = property on="Array" class="Arr (strict)"("Value"=w353) -> ()  [unwired: 2 in, 2 out]
    }
  }
  n189 = property on="Array" class="Arr (strict)"(error in=w20) -> ("Value"=w11:string[])  [unwired: 1 in, 2 out]
  n190 = property on="Commutator" class="Bool (strict)"() -> ("Value"=w10:bool)  [unwired: 2 in, 2 out]
  n191 = case shown="True" w10 {
    tunnel: w11 -> [w363 w370]
    tunnel: [w362 w370] -> w8
    frame True {
      n192 = for {
        tunnel: [w369] -> w366 mode=indexing
        tunnel: w363 -> [w367] mode=indexing
        n193 = Concatenate Strings("c", w367) -> (w369:string)
      }
      n194 = Array Subset(array=w366, index=1) -> (w364:string[])  [unwired: 1 in]
      n195 = Build Array (concatenate)(w363, w364) -> (w362:string[])
    }
    frame False {
    }
  }
  n196 = property on="Comments" class="Arr (strict)"() -> ("Value"=w4:string[])  [unwired: 2 in, 2 out]
  n197 = for {
    tunnel: w8 -> [w373] mode=indexing
    shift-right: [w371] -> w6
    shift-left: "" -> [w372]
    n198 = Concatenate Strings(w372, w373, "\t") -> (w371:string)
  }
  n199 = for {
    tunnel: w4 -> [w377] mode=indexing
    shift-right: [w375] -> w3
    shift-left: "" -> [w376]
    n200 = Concatenate Strings(w376, w377, "\t") -> (w375:string)
  }
  n201 = property on="Ring" class="Ring (strict)"("Strings []"=w8) -> (error out=w9:errorcluster)  [unwired: 2 in, 1 out]
  n202 = property on="Data file:" class="Path"(error in=w9) -> (error out=w17:errorcluster, "Value"=w19:path)  [unwired: 1 in, 1 out]
  n203 = while {
    tunnel: w17 -> [w392]
    shift-right: [w389] -> w16
    shift-left: dbl[][] [] -> [w391]
    shift-right: [w381] -> _
    shift-left: w12 -> [w388]
    tunnel: "points at each Vg" -> [w383]
    tunnel: [w379] -> w14
    stop <- w390 stop-if-true
    w379 = 1e-08
    # "send new Vg value to main Keithley 2400"
    n204 = for {
      N: w383 -> [_]
      tunnel: w392 -> [w408]
      tunnel: [w426] -> w390
      shift-right: [w413] -> w389
      shift-left: w391 -> [w439]
      tunnel: w388 -> [w424]
      tunnel: [w431] -> w381
      w425 = dbl[] []  # Empty array for data
      # "this part appends last\nmeasured point to the \ndata file"
      # "this line is current gate voltage"
      # "First we create an empty array \nfor data and write the first element \ninto it - current gate voltage"
      # "time is measured at the beginning\nand at the end of the cycle to\ncalculate delay time required to\nkeep set sweep rate"
      # "this part calculate resistances and current (if needed) from voltages measured by lock-in amplifiers"
      # "check if the next step doesn't\ngo beyond the target voltage"
      # "calculate difference between target and current Vg"
      # "check if we are at the target voltage yet"
      # "in this part we calculate incriment for Vg"
      n205 = flat-sequence {
        tunnel: w408 -> [w1613]
        tunnel: [w1613] -> w406
        tunnel: [w1615] -> w407
        tunnel: w406 -> [w1615]
        tunnel: [w1614] -> w405
        frame #0 {
          n206 = property on="Deliberate Time delay" class="DigNum (strict)"() -> ("Value"=w1612:i32)  [unwired: 2 in, 2 out]
          n207 = Wait (ms)(milliseconds to wait=w1612) -> ()  [unwired: 1 out]
        }
        frame #1 {
          n208 = Tick Count (ms)() -> (millisecond timer value=w1614:u32)
        }
      }
      n209 = Build Array (concatenate)(w425, w424) -> (w423:dbl[])
      n210 = property on="array for data" class="Arr (strict)"(error in=w407, "Value"=w423) -> (error out=w422:errorcluster)  [unwired: 1 in, 1 out]
      n211 = case shown="False" "Commutator" {
        tunnel: [w466 w1246] -> w440
        tunnel: w422 -> [w467 w1245]
        frame True {
          n212 = stacked-sequence {
            tunnel: w467 -> [w484 w873]
            tunnel: [_ w858] -> w466
            frame #0 {
              n213 = stacked-sequence {
                tunnel: w484 -> [w488 _ _ _ _ _ _ _ _ _ _ _ _ _ _ _ _ _ _ _ _ _ _ _ _ _]
                tunnel: [w488 _ _ _ _ _ _ _ _ _ _ _ _ _ _ _ _ _ _ _ _ _ _ _ _ _] -> w468
                frame #0 {
                  # "check if oscillator on \nlock-in (address 1)\nis to be measured"
                  n214 = property on="Current is:" class="RadioBtnsControl (strict)"() -> ("Value"=w491:T1)  [unwired: 2 in, 2 out]
                  n215 = property on="array for data" class="Arr (strict)"() -> ("Value"=w490:dbl[])  [unwired: 2 in, 2 out]
                  n216 = Equal?(x=w491, y=1) -> (x = y?=w492:bool)
                  n217 = case shown="False" w492 {
                    tunnel: w490 -> [w494 w502]
                    tunnel: [w494 w501] -> w489
                    frame False {
                      # "we are not measuring oscillator from\nlock-in (address 1)"
                    }
                    frame True {
                      w498 = "1"
                      # "we are  measuring oscillator"
                      n218 = GPIB Write(0:w498, 1:"SLVL?") -> (6:w499:errorcluster)  [unwired: 3 in, 1 out]
                      n219 = GPIB Read(0:w498, 1:3200, 3:w499) -> (5:w496:string)  [unwired: 2 in, 2 out]
                      n220 = Fract/Exp String To Number(string=w496) -> (number=w495:dbl)  [unwired: 3 in, 1 out]
                      n221 = Build Array (concatenate)(w502, w495) -> (w501:dbl[])
                    }
                  }
                  n222 = property on="array for data" class="Arr (strict)"("Value"=w489) -> ()  [unwired: 2 in, 2 out]
                }
                frame #1 {
                  # "check if in-phase\nsignal on lock-in \n(address 1) is to\nbe measured"
                  n223 = property on="array for data" class="Arr (strict)"() -> ("Value"=w505:dbl[])  [unwired: 2 in, 2 out]
                  n224 = property on="Addr 1 lock-in" class="Bool (strict)"() -> ("Value"=w503:bool)  [unwired: 2 in, 2 out]
                  n225 = case shown="False" w503 {
                    tunnel: w505 -> [w506 w514]
                    tunnel: [w506 w513] -> w504
                    frame False {
                      # "we are not measuring in phase signal on lock-in (address 1)"
                    }
                    frame True {
                      w511 = "1"
                      # "we are  measuring lock-in (address 1), in phase"
                      n226 = GPIB Write(0:w511, 1:"OUTP?1") -> (6:w512:errorcluster)  [unwired: 3 in, 1 out]
                      n227 = GPIB Read(0:w511, 1:3200, 3:w512) -> (5:w509:string)  [unwired: 2 in, 2 out]
                      n228 = Fract/Exp String To Number(string=w509) -> (number=w508:dbl)  [unwired: 3 in, 1 out]
                      n229 = Build Array (concatenate)(w514, w508) -> (w513:dbl[])
                    }
                  }
                  n230 = property on="array for data" class="Arr (strict)"("Value"=w504) -> ()  [unwired: 2 in, 2 out]
                }
                frame #2 {
                  # "check if out-of-phase\nsignal on lock-in \n(address 1) is to\nbe measured"
                  n231 = property on="Addr 1 lock-in oop" class="Bool (strict)"() -> ("Value"=w515:bool)  [unwired: 2 in, 2 out]
                  n232 = property on="array for data" class="Arr (strict)"() -> ("Value"=w517:dbl[])  [unwired: 2 in, 2 out]
                  n233 = case shown="False" w515 {
                    tunnel: w517 -> [w518 w526]
                    tunnel: [w518 w525] -> w516
                    frame False {
                      # "we are not measuring out-of-phase signal on lock-in (address 1)"
                    }
                    frame True {
                      w523 = "1"
                      # "we are  measuring lock-in (address 1), out-of-phase signal"
                      n234 = GPIB Write(0:w523, 1:"OUTP?2") -> (6:w524:errorcluster)  [unwired: 3 in, 1 out]
                      n235 = GPIB Read(0:w523, 1:3200, 3:w524) -> (5:w521:string)  [unwired: 2 in, 2 out]
                      n236 = Fract/Exp String To Number(string=w521) -> (number=w520:dbl)  [unwired: 3 in, 1 out]
                      n237 = Build Array (concatenate)(w526, w520) -> (w525:dbl[])
                    }
                  }
                  n238 = property on="array for data" class="Arr (strict)"("Value"=w516) -> ()  [unwired: 2 in, 2 out]
                }
                frame #3 {
                  # "check if in-phase\nsignal on lock-in \n(address 2) is to\nbe measured"
                  n239 = property on="Addr 2 lock-in" class="Bool (strict)"() -> ("Value"=w527:bool)  [unwired: 2 in, 2 out]
                  n240 = property on="array for data" class="Arr (strict)"() -> ("Value"=w529:dbl[])  [unwired: 2 in, 2 out]
                  n241 = case shown="False" w527 {
                    tunnel: w529 -> [w530 w538]
                    tunnel: [w530 w537] -> w528
                    frame False {
                      # "we are not measuring in phase signal on lock-in (address 2)"
                    }
                    frame True {
                      w535 = "2"
                      # "we are  measuring lock-in (address 2), in phase"
                      n242 = GPIB Write(0:w535, 1:"OUTP?1") -> (6:w536:errorcluster)  [unwired: 3 in, 1 out]
                      n243 = GPIB Read(0:w535, 1:3200, 3:w536) -> (5:w533:string)  [unwired: 2 in, 2 out]
                      n244 = Fract/Exp String To Number(string=w533) -> (number=w532:dbl)  [unwired: 3 in, 1 out]
                      n245 = Build Array (concatenate)(w538, w532) -> (w537:dbl[])
                    }
                  }
                  n246 = property on="array for data" class="Arr (strict)"("Value"=w528) -> ()  [unwired: 2 in, 2 out]
                }
                frame #4 {
                  # "check if out-of-phase\nsignal on lock-in \n(address 2) is to\nbe measured"
                  n247 = property on="Addr 2 lock-in oop" class="Bool (strict)"() -> ("Value"=w539:bool)  [unwired: 2 in, 2 out]
                  n248 = property on="array for data" class="Arr (strict)"() -> ("Value"=w541:dbl[])  [unwired: 2 in, 2 out]
                  n249 = case shown="False" w539 {
                    tunnel: w541 -> [w542 w550]
                    tunnel: [w542 w549] -> w540
                    tunnel: w539 -> [_ _]
                    frame False {
                      # "we are not measuring out-of-phase signal on lock-in (address 2)"
                    }
                    frame True {
                      w547 = "2"
                      # "we are  measuring lock-in (address 2), out-of-phase"
                      n250 = GPIB Write(0:w547, 1:"OUTP?2") -> (6:w548:errorcluster)  [unwired: 3 in, 1 out]
                      n251 = GPIB Read(0:w547, 1:3200, 3:w548) -> (5:w545:string)  [unwired: 2 in, 2 out]
                      n252 = Fract/Exp String To Number(string=w545) -> (number=w544:dbl)  [unwired: 3 in, 1 out]
                      n253 = Build Array (concatenate)(w550, w544) -> (w549:dbl[])
                    }
                  }
                  n254 = property on="array for data" class="Arr (strict)"("Value"=w540) -> ()  [unwired: 2 in, 2 out]
                }
                frame #5 {
                  # "check if in-phase\nsignal on lock-in \n(address 3) is to\nbe measured"
                  n255 = property on="Addr 3 lock-in" class="Bool (strict)"() -> ("Value"=w551:bool)  [unwired: 2 in, 2 out]
                  n256 = property on="array for data" class="Arr (strict)"() -> ("Value"=w553:dbl[])  [unwired: 2 in, 2 out]
                  n257 = case shown="False" w551 {
                    tunnel: w553 -> [w554 w562]
                    tunnel: [w554 w561] -> w552
                    frame False {
                      # "we are not measuring in phase signal on lock-in (address 3)"
                    }
                    frame True {
                      w559 = "3"
                      # "we are  measuring lock-in (address 3), in phase"
                      n258 = GPIB Write(0:w559, 1:"OUTP?1") -> (6:w560:errorcluster)  [unwired: 3 in, 1 out]
                      n259 = GPIB Read(0:w559, 1:3200, 3:w560) -> (5:w557:string)  [unwired: 2 in, 2 out]
                      n260 = Fract/Exp String To Number(string=w557) -> (number=w556:dbl)  [unwired: 3 in, 1 out]
                      n261 = Build Array (concatenate)(w562, w556) -> (w561:dbl[])
                    }
                  }
                  n262 = property on="array for data" class="Arr (strict)"("Value"=w552) -> ()  [unwired: 2 in, 2 out]
                }
                frame #6 {
                  # "check if out-of-phase\nsignal on lock-in \n(address 3) is to\nbe measured"
                  n263 = property on="Addr 3 lock-in oop" class="Bool (strict)"() -> ("Value"=w563:bool)  [unwired: 2 in, 2 out]
                  n264 = property on="array for data" class="Arr (strict)"() -> ("Value"=w565:dbl[])  [unwired: 2 in, 2 out]
                  n265 = case shown="False" w563 {
                    tunnel: w565 -> [w566 w574]
                    tunnel: [w566 w573] -> w564
                    frame False {
                      # "we are not measuring out-of-phase signal on lock-in (address 3)"
                    }
                    frame True {
                      w571 = "3"
                      # "we are  measuring lock-in (address 3), out-of-phase"
                      n266 = GPIB Write(0:w571, 1:"OUTP?2") -> (6:w572:errorcluster)  [unwired: 3 in, 1 out]
                      n267 = GPIB Read(0:w571, 1:3200, 3:w572) -> (5:w569:string)  [unwired: 2 in, 2 out]
                      n268 = Fract/Exp String To Number(string=w569) -> (number=w568:dbl)  [unwired: 3 in, 1 out]
                      n269 = Build Array (concatenate)(w574, w568) -> (w573:dbl[])
                    }
                  }
                  n270 = property on="array for data" class="Arr (strict)"("Value"=w564) -> ()  [unwired: 2 in, 2 out]
                }
                frame #7 {
                  # "check if in-phase\nsignal on lock-in \n(address 4) is to\nbe measured"
                  n271 = property on="Addr 4 lock-in" class="Bool (strict)"() -> ("Value"=w575:bool)  [unwired: 2 in, 2 out]
                  n272 = property on="array for data" class="Arr (strict)"() -> ("Value"=w577:dbl[])  [unwired: 2 in, 2 out]
                  n273 = case shown="False" w575 {
                    tunnel: w577 -> [w578 w586]
                    tunnel: [w578 w585] -> w576
                    frame False {
                      # "we are not measuring in phase signal on lock-in (address 4)"
                    }
                    frame True {
                      w583 = "4"
                      # "we are  measuring lock-in (address 4), in phase"
                      n274 = GPIB Write(0:w583, 1:"OUTP?1") -> (6:w584:errorcluster)  [unwired: 3 in, 1 out]
                      n275 = GPIB Read(0:w583, 1:3200, 3:w584) -> (5:w581:string)  [unwired: 2 in, 2 out]
                      n276 = Fract/Exp String To Number(string=w581) -> (number=w580:dbl)  [unwired: 3 in, 1 out]
                      n277 = Build Array (concatenate)(w586, w580) -> (w585:dbl[])
                    }
                  }
                  n278 = property on="array for data" class="Arr (strict)"("Value"=w576) -> ()  [unwired: 2 in, 2 out]
                }
                frame #8 {
                  # "check if out-of-phase\nsignal on lock-in \n(address 4) is to\nbe measured"
                  n279 = property on="Addr 4 lock-in oop" class="Bool (strict)"() -> ("Value"=w587:bool)  [unwired: 2 in, 2 out]
                  n280 = property on="array for data" class="Arr (strict)"() -> ("Value"=w589:dbl[])  [unwired: 2 in, 2 out]
                  n281 = case shown="False" w587 {
                    tunnel: w589 -> [w590 w598]
                    tunnel: [w590 w597] -> w588
                    frame False {
                      # "we are not measuring out-of-phase signal on lock-in (address 4)"
                    }
                    frame True {
                      w595 = "4"
                      # "we are  measuring lock-in (address 4), out-of-phase"
                      n282 = GPIB Write(0:w595, 1:"OUTP?2") -> (6:w596:errorcluster)  [unwired: 3 in, 1 out]
                      n283 = GPIB Read(0:w595, 1:3200, 3:w596) -> (5:w593:string)  [unwired: 2 in, 2 out]
                      n284 = Fract/Exp String To Number(string=w593) -> (number=w592:dbl)  [unwired: 3 in, 1 out]
                      n285 = Build Array (concatenate)(w598, w592) -> (w597:dbl[])
                    }
                  }
                  n286 = property on="array for data" class="Arr (strict)"("Value"=w588) -> ()  [unwired: 2 in, 2 out]
                }
                frame #9 {
                  # "check if in-phase\nsignal on lock-in \n(address 5) is to\nbe measured"
                  n287 = property on="Addr 5 lock-in" class="Bool (strict)"() -> ("Value"=w599:bool)  [unwired: 2 in, 2 out]
                  n288 = property on="array for data" class="Arr (strict)"() -> ("Value"=w601:dbl[])  [unwired: 2 in, 2 out]
                  n289 = case shown="False" w599 {
                    tunnel: w601 -> [w602 w610]
                    tunnel: [w602 w609] -> w600
                    frame False {
                      # "we are not measuring in phase signal on lock-in (address 5)"
                    }
                    frame True {
                      w607 = "5"
                      # "we are  measuring lock-in (address 5), in phase"
                      n290 = GPIB Write(0:w607, 1:"OUTP?1") -> (6:w608:errorcluster)  [unwired: 3 in, 1 out]
                      n291 = GPIB Read(0:w607, 1:3200, 3:w608) -> (5:w605:string)  [unwired: 2 in, 2 out]
                      n292 = Fract/Exp String To Number(string=w605) -> (number=w604:dbl)  [unwired: 3 in, 1 out]
                      n293 = Build Array (concatenate)(w610, w604) -> (w609:dbl[])
                    }
                  }
                  n294 = property on="array for data" class="Arr (strict)"("Value"=w600) -> ()  [unwired: 2 in, 2 out]
                }
                frame #10 {
                  # "check if out-of-phase\nsignal on lock-in \n(address 5) is to\nbe measured"
                  n295 = property on="Addr 5 lock-in oop" class="Bool (strict)"() -> ("Value"=w611:bool)  [unwired: 2 in, 2 out]
                  n296 = property on="array for data" class="Arr (strict)"() -> ("Value"=w613:dbl[])  [unwired: 2 in, 2 out]
                  n297 = case shown="False" w611 {
                    tunnel: w613 -> [w614 w622]
                    tunnel: [w614 w621] -> w612
                    frame False {
                      # "we are not measuring out-of-phase signal on lock-in (address 5)"
                    }
                    frame True {
                      w619 = "5"
                      # "we are  measuring lock-in (address 5), out-of-phase"
                      n298 = GPIB Write(0:w619, 1:"OUTP?2") -> (6:w620:errorcluster)  [unwired: 3 in, 1 out]
                      n299 = GPIB Read(0:w619, 1:3200, 3:w620) -> (5:w617:string)  [unwired: 2 in, 2 out]
                      n300 = Fract/Exp String To Number(string=w617) -> (number=w616:dbl)  [unwired: 3 in, 1 out]
                      n301 = Build Array (concatenate)(w622, w616) -> (w621:dbl[])
                    }
                  }
                  n302 = property on="array for data" class="Arr (strict)"("Value"=w612) -> ()  [unwired: 2 in, 2 out]
                }
                frame #11 {
                  # "check if voltage on \nmain Keithley 2400 \n(addr. 12) is to\nbe measured"
                  n303 = property on="Voltage (Vk1)" class="Bool (strict)"() -> ("Value"=w623:bool)  [unwired: 2 in, 2 out]
                  n304 = property on="array for data" class="Arr (strict)"() -> ("Value"=w625:dbl[])  [unwired: 2 in, 2 out]
                  n305 = case shown="False" w623 {
                    tunnel: w625 -> [w626 w636]
                    tunnel: [w626 w635] -> w624
                    frame False {
                      # "we aren't measuring voltage \non main Keithley 2400 (addr. 12)"
                    }
                    frame True {
                      w633 = "12"
                      # "we are measuring voltage \non main Keithley 2400 (addr. 12)"
                      n306 = GPIB Write(0:w633, 1:":READ?") -> (6:w634:errorcluster)  [unwired: 3 in, 1 out]
                      n307 = GPIB Read(0:w633, 1:3200, 3:w634) -> (5:w629:string)  [unwired: 2 in, 2 out]
                      n308 = String Subset(string=w629, length (rest)=13) -> (substring=w628:string)  [unwired: 1 in]
                      n309 = Fract/Exp String To Number(string=w628) -> (number=w631:dbl)  [unwired: 3 in, 1 out]
                      n310 = Build Array (concatenate)(w636, w631) -> (w635:dbl[])
                    }
                  }
                  n311 = property on="array for data" class="Arr (strict)"("Value"=w624) -> ()  [unwired: 2 in, 2 out]
                }
                frame #12 {
                  # "check if  current on \nmain Keithley 2400 \n(addr. 12) is to\nbe measured"
                  n312 = property on="Current (Ik1)" class="Bool (strict)"() -> ("Value"=w637:bool)  [unwired: 2 in, 2 out]
                  n313 = property on="array for data" class="Arr (strict)"() -> ("Value"=w639:dbl[])  [unwired: 2 in, 2 out]
                  n314 = case shown="True" w637 {
                    tunnel: w639 -> [w640 w651]
                    tunnel: [w640 w650] -> w638
                    frame False {
                      # "we aren't measuring current \non main Keithley 2400 (addr. 12)"
                    }
                    frame True {
                      w648 = "12"
                      # "we are measuring current\non main Keithley 2400 (addr. 12)"
                      n315 = GPIB Write(0:w648, 1:":READ?") -> (6:w649:errorcluster)  [unwired: 3 in, 1 out]
                      n316 = GPIB Read(0:w648, 1:3200, 3:w649) -> (5:w644:string)  [unwired: 2 in, 2 out]
                      n317 = String Subset(string=w644, offset (0)=14, length (rest)=13) -> (substring=w643:string)
                      n318 = Fract/Exp String To Number(string=w643) -> (number=w646:dbl)  [unwired: 3 in, 1 out]
                      n319 = Build Array (concatenate)(w651, w646) -> (w650:dbl[])
                    }
                  }
                  n320 = property on="array for data" class="Arr (strict)"("Value"=w638) -> ()  [unwired: 2 in, 2 out]
                }
                frame #13 {
                  # "check if voltage on \nadd. Keithley 2400 \n(addr. 13) is to\nbe measured"
                  n321 = property on="Voltage (Vk2)" class="Bool (strict)"() -> ("Value"=w652:bool)  [unwired: 2 in, 2 out]
                  n322 = property on="array for data" class="Arr (strict)"() -> ("Value"=w654:dbl[])  [unwired: 2 in, 2 out]
                  n323 = case shown="True" w652 {
                    tunnel: w654 -> [w655 w665]
                    tunnel: [w655 w664] -> w653
                    frame False {
                      # "we aren't measuring voltage \non additional Keithley 2400 (addr. 13)"
                    }
                    frame True {
                      w662 = "13"
                      # "we are measuring voltage \non additional Keithley 2400 (addr. 13)"
                      n324 = GPIB Write(0:w662, 1:":READ?") -> (6:w663:errorcluster)  [unwired: 3 in, 1 out]
                      n325 = GPIB Read(0:w662, 1:3200, 3:w663) -> (5:w658:string)  [unwired: 2 in, 2 out]
                      n326 = String Subset(string=w658, length (rest)=13) -> (substring=w657:string)  [unwired: 1 in]
                      n327 = Fract/Exp String To Number(string=w657) -> (number=w660:dbl)  [unwired: 3 in, 1 out]
                      n328 = Build Array (concatenate)(w665, w660) -> (w664:dbl[])
                    }
                  }
                  n329 = property on="array for data" class="Arr (strict)"("Value"=w653) -> ()  [unwired: 2 in, 2 out]
                }
                frame #14 {
                  # "check if  current on \nadd. Keithley 2400 \n(addr. 13) is to\nbe measured"
                  n330 = property on="Current (Ik2)" class="Bool (strict)"() -> ("Value"=w666:bool)  [unwired: 2 in, 2 out]
                  n331 = property on="array for data" class="Arr (strict)"() -> ("Value"=w668:dbl[])  [unwired: 2 in, 2 out]
                  n332 = case shown="True" w666 {
                    tunnel: w668 -> [w669 w680]
                    tunnel: [w669 w679] -> w667
                    frame False {
                      # "we aren't measuring current \non additional Keithley 2400 (addr. 13)"
                    }
                    frame True {
                      w677 = "13"
                      # "we are measuring current\non additional Keithley 2400 (addr. 13)"
                      n333 = GPIB Write(0:w677, 1:":READ?") -> (6:w678:errorcluster)  [unwired: 3 in, 1 out]
                      n334 = GPIB Read(0:w677, 1:3200, 3:w678) -> (5:w673:string)  [unwired: 2 in, 2 out]
                      n335 = String Subset(string=w673, offset (0)=14, length (rest)=13) -> (substring=w672:string)
                      n336 = Fract/Exp String To Number(string=w672) -> (number=w675:dbl)  [unwired: 3 in, 1 out]
                      n337 = Build Array (concatenate)(w680, w675) -> (w679:dbl[])
                    }
                  }
                  n338 = property on="array for data" class="Arr (strict)"("Value"=w667) -> ()  [unwired: 2 in, 2 out]
                }
                frame #15 {
                  # "check if voltage on \nadd. Keithley 2400 \n(addr. 14) is to\nbe measured"
                  n339 = property on="Voltage (Vk3)" class="Bool (strict)"() -> ("Value"=w681:bool)  [unwired: 2 in, 2 out]
                  n340 = property on="array for data" class="Arr (strict)"() -> ("Value"=w683:dbl[])  [unwired: 2 in, 2 out]
                  n341 = case shown="True" w681 {
                    tunnel: w683 -> [w684 w694]
                    tunnel: [w684 w693] -> w682
                    frame False {
                      # "we aren't measuring voltage \non additional Keithley 2400 (addr. 14)"
                    }
                    frame True {
                      w691 = "14"
                      # "we are measuring voltage \non additional Keithley 2400 (addr. 14)"
                      n342 = GPIB Write(0:w691, 1:":READ?") -> (6:w692:errorcluster)  [unwired: 3 in, 1 out]
                      n343 = GPIB Read(0:w691, 1:3200, 3:w692) -> (5:w687:string)  [unwired: 2 in, 2 out]
                      n344 = String Subset(string=w687, length (rest)=13) -> (substring=w686:string)  [unwired: 1 in]
                      n345 = Fract/Exp String To Number(string=w686) -> (number=w689:dbl)  [unwired: 3 in, 1 out]
                      n346 = Build Array (concatenate)(w694, w689) -> (w693:dbl[])
                    }
                  }
                  n347 = property on="array for data" class="Arr (strict)"("Value"=w682) -> ()  [unwired: 2 in, 2 out]
                }
                frame #16 {
                  # "check if  current on \nadd. Keithley 2400 \n(addr. 14) is to\nbe measured"
                  n348 = property on="Current (Ik3)" class="Bool (strict)"() -> ("Value"=w695:bool)  [unwired: 2 in, 2 out]
                  n349 = property on="array for data" class="Arr (strict)"() -> ("Value"=w697:dbl[])  [unwired: 2 in, 2 out]
                  n350 = case shown="True" w695 {
                    tunnel: w697 -> [w698 w709]
                    tunnel: [w698 w708] -> w696
                    frame False {
                      # "we aren't measuring current \non additional Keithley 2400 (addr. 14)"
                    }
                    frame True {
                      w706 = "14"
                      # "we are measuring current\non additional Keithley 2400 (addr. 14)"
                      n351 = GPIB Write(0:w706, 1:":READ?") -> (6:w707:errorcluster)  [unwired: 3 in, 1 out]
                      n352 = GPIB Read(0:w706, 1:3200, 3:w707) -> (5:w702:string)  [unwired: 2 in, 2 out]
                      n353 = String Subset(string=w702, offset (0)=14, length (rest)=13) -> (substring=w701:string)
                      n354 = Fract/Exp String To Number(string=w701) -> (number=w704:dbl)  [unwired: 3 in, 1 out]
                      n355 = Build Array (concatenate)(w709, w704) -> (w708:dbl[])
                    }
                  }
                  n356 = property on="array for data" class="Arr (strict)"("Value"=w696) -> ()  [unwired: 2 in, 2 out]
                }
                frame #17 {
                  # "check if 1st channel\non Keithley 2182 \n(addr. 15) is to\nbe measured"
                  n357 = property on="Channel 1 (Vnano1)" class="Bool (strict)"() -> ("Value"=w710:bool)  [unwired: 2 in, 2 out]
                  n358 = property on="array for data" class="Arr (strict)"() -> ("Value"=w712:dbl[])  [unwired: 2 in, 2 out]
                  n359 = case shown="True" w710 {
                    tunnel: w712 -> [w713 w721]
                    tunnel: [w713 w720] -> w711
                    frame False {
                      # "we are not measuring 1st channel\non Keithley 2182 (addr. 15)"
                    }
                    frame True {
                      w718 = "15"
                      # "we are measuring 1st channel\non Keithley 2182 (addr. 15)"
                      n360 = GPIB Write(0:w718, 1:":SENSe:DATA:FRES?") -> (6:w719:errorcluster)  [unwired: 3 in, 1 out]
                      n361 = GPIB Read(0:w718, 1:200, 3:w719) -> (5:w714:string)  [unwired: 2 in, 2 out]
                      n362 = Fract/Exp String To Number(string=w714) -> (number=w716:dbl)  [unwired: 3 in, 1 out]
                      n363 = Build Array (concatenate)(w721, w716) -> (w720:dbl[])
                    }
                  }
                  n364 = property on="array for data" class="Arr (strict)"("Value"=w711) -> ()  [unwired: 2 in, 2 out]
                }
                frame #18 {
                  # "check if 2nd channel\non Keithley 2182 \n(addr. 15) is to\nbe measured"
                  n365 = property on="Channel 2 (Vnano1b)" class="Bool (strict)"() -> ("Value"=w722:bool)  [unwired: 2 in, 2 out]
                  n366 = property on="array for data" class="Arr (strict)"() -> ("Value"=w724:dbl[])  [unwired: 2 in, 2 out]
                  n367 = case shown="False" w722 {
                    tunnel: w724 -> [w725 w737]
                    tunnel: [w725 w736] -> w723
                    frame False {
                      # "we are not measuring 1st channel\non Keithley 2182 (addr. 15)"
                    }
                    frame True {
                      w728 = "15"
                      # "switching to channel 2 and then\nback to channel 1"
                      # "we are measuring 2nd channel\non Keithley 2182 (addr. 15)"
                      n368 = GPIB Write(0:w728, 1:":SENSe:CHAN 2") -> (6:w729:errorcluster)  [unwired: 3 in, 1 out]
                      n369 = GPIB Write(0:w728, 1:":SENSe:DATA:FRES?", 3:w729) -> (6:w735:errorcluster)  [unwired: 2 in, 1 out]
                      n370 = GPIB Read(0:w728, 1:200, 3:w735) -> (5:w731:string, 7:w727:errorcluster)  [unwired: 2 in, 1 out]
                      n371 = GPIB Write(0:w728, 1:":SENSe:CHAN 1", 3:w727) -> ()  [unwired: 2 in, 2 out]
                      n372 = Fract/Exp String To Number(string=w731) -> (number=w733:dbl)  [unwired: 3 in, 1 out]
                      n373 = Build Array (concatenate)(w737, w733) -> (w736:dbl[])
                    }
                  }
                  n374 = property on="array for data" class="Arr (strict)"("Value"=w723) -> ()  [unwired: 2 in, 2 out]
                }
                frame #19 {
                  # "check if 1st channel\non Keithley 2182 \n(addr. 16) is to\nbe measured"
                  n375 = property on="Channel 1 (Vnano2)" class="Bool (strict)"() -> ("Value"=w738:bool)  [unwired: 2 in, 2 out]
                  n376 = property on="array for data" class="Arr (strict)"() -> ("Value"=w740:dbl[])  [unwired: 2 in, 2 out]
                  n377 = case shown="True" w738 {
                    tunnel: w740 -> [w741 w749]
                    tunnel: [w741 w748] -> w739
                    frame False {
                      # "we are not measuring 1st channel\non Keithley 2182 (addr. 16)"
                    }
                    frame True {
                      w746 = "16"
                      # "we are measuring 1st channel\non Keithley 2182 (addr. 16)"
                      n378 = GPIB Write(0:w746, 1:":SENSe:DATA:FRES?") -> (6:w747:errorcluster)  [unwired: 3 in, 1 out]
                      n379 = GPIB Read(0:w746, 1:200, 3:w747) -> (5:w742:string)  [unwired: 2 in, 2 out]
                      n380 = Fract/Exp String To Number(string=w742) -> (number=w744:dbl)  [unwired: 3 in, 1 out]
                      n381 = Build Array (concatenate)(w749, w744) -> (w748:dbl[])
                    }
                  }
                  n382 = property on="array for data" class="Arr (strict)"("Value"=w739) -> ()  [unwired: 2 in, 2 out]
                }
                frame #20 {
                  # "check if 2nd channel\non Keithley 2182 \n(addr. 16) is to\nbe measured"
                  n383 = property on="Channel 2 (Vnano2b)" class="Bool (strict)"() -> ("Value"=w750:bool)  [unwired: 2 in, 2 out]
                  n384 = property on="array for data" class="Arr (strict)"() -> ("Value"=w752:dbl[])  [unwired: 2 in, 2 out]
                  n385 = case shown="False" w750 {
                    tunnel: w752 -> [w753 w765]
                    tunnel: [w753 w764] -> w751
                    frame False {
                      # "we are not measuring 1st channel\non Keithley 2182 (addr. 16)"
                    }
                    frame True {
                      w756 = "16"
                      # "switching to channel 2 and then\nback to channel 1"
                      # "we are measuring 2nd channel\non Keithley 2182 (addr. 16)"
                      n386 = GPIB Write(0:w756, 1:":SENSe:CHAN 2") -> (6:w757:errorcluster)  [unwired: 3 in, 1 out]
                      n387 = GPIB Write(0:w756, 1:":SENSe:DATA:FRES?", 3:w757) -> (6:w763:errorcluster)  [unwired: 2 in, 1 out]
                      n388 = GPIB Read(0:w756, 1:200, 3:w763) -> (5:w759:string, 7:w755:errorcluster)  [unwired: 2 in, 1 out]
                      n389 = GPIB Write(0:w756, 1:":SENSe:CHAN 1", 3:w755) -> ()  [unwired: 2 in, 2 out]
                      n390 = Fract/Exp String To Number(string=w759) -> (number=w761:dbl)  [unwired: 3 in, 1 out]
                      n391 = Build Array (concatenate)(w765, w761) -> (w764:dbl[])
                    }
                  }
                  n392 = property on="array for data" class="Arr (strict)"("Value"=w751) -> ()  [unwired: 2 in, 2 out]
                }
                frame #21 {
                  # "check if 1st channel\non Keithley 2182 \n(addr. 17) is to\nbe measured"
                  n393 = property on="Channel 1 (Vnano3)" class="Bool (strict)"() -> ("Value"=w766:bool)  [unwired: 2 in, 2 out]
                  n394 = property on="array for data" class="Arr (strict)"() -> ("Value"=w768:dbl[])  [unwired: 2 in, 2 out]
                  n395 = case shown="True" w766 {
                    tunnel: w768 -> [w769 w777]
                    tunnel: [w769 w776] -> w767
                    frame False {
                      # "we are not measuring 1st channel\non Keithley 2182 (addr. 17)"
                    }
                    frame True {
                      w774 = "17"
                      # "we are measuring 1st channel\non Keithley 2182 (addr. 17)"
                      n396 = GPIB Write(0:w774, 1:":SENSe:DATA:FRES?") -> (6:w775:errorcluster)  [unwired: 3 in, 1 out]
                      n397 = GPIB Read(0:w774, 1:200, 3:w775) -> (5:w770:string)  [unwired: 2 in, 2 out]
                      n398 = Fract/Exp String To Number(string=w770) -> (number=w772:dbl)  [unwired: 3 in, 1 out]
                      n399 = Build Array (concatenate)(w777, w772) -> (w776:dbl[])
                    }
                  }
                  n400 = property on="array for data" class="Arr (strict)"("Value"=w767) -> ()  [unwired: 2 in, 2 out]
                }
                frame #22 {
                  # "check if 2nd channel\non Keithley 2182 \n(addr. 17) is to\nbe measured"
                  n401 = property on="Channel 2 (Vnano3b)" class="Bool (strict)"() -> ("Value"=w778:bool)  [unwired: 2 in, 2 out]
                  n402 = property on="array for data" class="Arr (strict)"() -> ("Value"=w780:dbl[])  [unwired: 2 in, 2 out]
                  n403 = case shown="False" w778 {
                    tunnel: w780 -> [w781 w793]
                    tunnel: [w781 w792] -> w779
                    frame False {
                      # "we are not measuring 1st channel\non Keithley 2182 (addr. 17)"
                    }
                    frame True {
                      w784 = "17"
                      # "switching to channel 2 and then\nback to channel 1"
                      # "we are measuring 2nd channel\non Keithley 2182 (addr. 17)"
                      n404 = GPIB Write(0:w784, 1:":SENSe:CHAN 2") -> (6:w785:errorcluster)  [unwired: 3 in, 1 out]
                      n405 = GPIB Write(0:w784, 1:":SENSe:DATA:FRES?", 3:w785) -> (6:w791:errorcluster)  [unwired: 2 in, 1 out]
                      n406 = GPIB Read(0:w784, 1:200, 3:w791) -> (5:w787:string, 7:w783:errorcluster)  [unwired: 2 in, 1 out]
                      n407 = GPIB Write(0:w784, 1:":SENSe:CHAN 1", 3:w783) -> ()  [unwired: 2 in, 2 out]
                      n408 = Fract/Exp String To Number(string=w787) -> (number=w789:dbl)  [unwired: 3 in, 1 out]
                      n409 = Build Array (concatenate)(w793, w789) -> (w792:dbl[])
                    }
                  }
                  n410 = property on="array for data" class="Arr (strict)"("Value"=w779) -> ()  [unwired: 2 in, 2 out]
                }
                frame #23 {
                  # "check if 1st \nthermometer on \nOxford ITC \n(address 24) \nis measured"
                  n411 = property on="Thermometer 1 (T1)" class="Bool (strict)"() -> ("Value"=w794:bool)  [unwired: 2 in, 2 out]
                  n412 = property on="array for data" class="Arr (strict)"() -> ("Value"=w796:dbl[])  [unwired: 2 in, 2 out]
                  n413 = case shown="True" w794 {
                    tunnel: w796 -> [w797 w806]
                    tunnel: [w797 w805] -> w795
                    frame False {
                      # "we are not measuring temperature on\nthermometer 1 (addr. 24)"
                    }
                    frame True {
                      w798 = 1
                      w803 = "24"
                      # "we are measuring temperature,\nthermometer 1 (addr. 24)"
                      n414 = GPIB Write(0:w803, 1:"R 1", 2:w798) -> (6:w804:errorcluster)  [unwired: 2 in, 1 out]
                      n415 = GPIB Read(0:w803, 1:200, 2:w798, 3:w804) -> (5:w799:string)  [unwired: 1 in, 2 out]
                      n416 = Fract/Exp String To Number(string=w799, offset=w798) -> (number=w801:dbl)  [unwired: 2 in, 1 out]
                      n417 = Build Array (concatenate)(w806, w801) -> (w805:dbl[])
                    }
                  }
                  n418 = property on="array for data" class="Arr (strict)"("Value"=w795) -> ()  [unwired: 2 in, 2 out]
                }
                frame #24 {
                  # "check if 1st \nthermometer on \nOxford ITC \n(address 24) \nis measured"
                  n419 = property on="Magnetic Field (B)" class="Bool (strict)"() -> ("Value"=w807:bool)  [unwired: 2 in, 2 out]
                  n420 = property on="array for data" class="Arr (strict)"() -> ("Value"=w809:dbl[])  [unwired: 2 in, 2 out]
                  n421 = case shown="True" w807 {
                    tunnel: w809 -> [w810 w819]
                    tunnel: [w810 w818] -> w808
                    frame False {
                      # "we are not measuringmagnetic field (addr. 25)"
                    }
                    frame True {
                      w811 = 1
                      w816 = "25"
                      # "we are measuring magnetic field  (addr. 25)"
                      n422 = GPIB Write(0:w816, 1:"R 7", 2:w811) -> (6:w817:errorcluster)  [unwired: 2 in, 1 out]
                      n423 = GPIB Read(0:w816, 1:200, 2:w811, 3:w817) -> (5:w812:string)  [unwired: 1 in, 2 out]
                      n424 = Fract/Exp String To Number(string=w812, offset=w811) -> (number=w814:dbl)  [unwired: 2 in, 1 out]
                      n425 = Build Array (concatenate)(w819, w814) -> (w818:dbl[])
                    }
                  }
                  n426 = property on="array for data" class="Arr (strict)"("Value"=w808) -> ()  [unwired: 2 in, 2 out]
                }
                frame #25 {
                  # "check if capacitance\nand loss (address 28)\nare measured"
                  n427 = property on="Capacitance (C) and Loss (L)" class="Bool (strict)"() -> ("Value"=w820:bool)  [unwired: 2 in, 2 out]
                  n428 = property on="array for data" class="Arr (strict)"() -> ("Value"=w822:dbl[])  [unwired: 2 in, 2 out]
                  n429 = case shown="False" w820 {
                    tunnel: w822 -> [w823 w829]
                    tunnel: [w823 w825] -> w821
                    frame False {
                      # "we are not measuringmagnetic capacitance (addr. 28)"
                    }
                    frame True {
                      # "we are measuring capacitance and loss  (addr. 28)"
                      n430 = stacked-sequence {
                        seq-local: [w831 _ _] -> [_ _ w854]
                        tunnel: [_ _ w848] -> w824
                        tunnel: [_ _ w849] -> w827
                        tunnel: "28" ("data") -> [w830 w834 w843]
                        frame #0 {
                          n431 = GPIB Write(0:w830, 1:"SINGLE" ("data"), 2:i16 0 ("mode (0)")) -> (6:w831:errorcluster)  [unwired: 2 in, 1 out]
                        }
                        frame #1 {
                          n432 = while {
                            tunnel: w834 -> [w835]
                            i -> [w836]
                            stop <- w838 continue-if-true
                            n433 = GPIB Serial Poll(0:w835) -> (2:w840:i16)  [unwired: 1 in, 2 out]
                            n434 = Less?(x=w840, y=i16 128) -> (x < y?=w838:bool)
                            n435 = Wait (ms)(milliseconds to wait=u32 50) -> ()  [unwired: 1 out]
                            "Numeric" <- w836
                          }
                        }
                        frame #2 {
                          w841 = i16 2 ("mode (0)")
                          n436 = GPIB Read(0:w843, 1:200 ("byte count"), 2:i16 2 ("mode (0)"), 3:w854) -> (5:w847:string)  [unwired: 1 in, 2 out]
                          n437 = Match Pattern(string=w847, regular expression="C=") -> (after substring=w846:string)  [unwired: 1 in, 3 out]
                          n438 = Match Pattern(string=w846, regular expression="PF L=") -> (after substring=w844:string)  [unwired: 1 in, 3 out]
                          n439 = Search/Split String(string=w846, search string/char (-)=" ", offset (0)=w841) -> (substring before match=w851:string)  [unwired: 2 out]
                          n440 = Search/Split String(string=w844, search string/char (-)=" ", offset (0)=w841) -> (substring before match=w850:string)  [unwired: 2 out]
                          n441 = Fract/Exp String To Number(string=w850) -> (number=w848:dbl)  [unwired: 3 in, 1 out]
                          n442 = Fract/Exp String To Number(string=w851) -> (number=w849:dbl)  [unwired: 3 in, 1 out]
                        }
                      }
                      n443 = Build Array (concatenate)(w829, w827) -> (w826:dbl[])
                      n444 = Build Array (concatenate)(w826, w824) -> (w825:dbl[])
                    }
                  }
                  n445 = property on="array for data" class="Arr (strict)"("Value"=w821) -> ()  [unwired: 2 in, 2 out]
                }
              }
              n446 = flat-sequence {
                tunnel: w469 -> [_]
                frame #0 {
                  n447 = property on="Delib Time delay" class="DigNum (strict)"() -> ("Value"=w485:i32)  [unwired: 2 in, 2 out]
                  n448 = Wait (ms)(milliseconds to wait=w485) -> ()  [unwired: 1 out]
                }
              }
              n449 = case shown="\"Radio Selection 2\"" "Commute SorceMeter" {
                tunnel: ["13" "14"] -> w470
                frame "Radio Selection 1", Default {
                }
                frame "Radio Selection 2" {
                }
              }
              n450 = GPIB Write(0:w470, 1:":READ?", 3:w468) -> (6:w471:errorcluster)  [unwired: 2 in, 1 out]
              n451 = GPIB Read(0:w470, 1:3200, 3:w471) -> (5:w474:string)  [unwired: 2 in, 2 out]
              n452 = String Subset(string=w474, length (rest)=13) -> (substring=w475:string)  [unwired: 1 in]
              n453 = Fract/Exp String To Number(string=w475) -> (number=w477:dbl)  [unwired: 3 in, 1 out]
              n454 = Multiply(x=w477, y=-1.0) -> (x*y=w482:dbl)
              n455 = Number To Fractional String(number=w482) -> (F-format string=w479:string)  [unwired: 3 in]
              n456 = Concatenate Strings(":INIT:IMM; :SOUR:VOLT:LEV:IMM:AMPL " ("data"), w479) -> (w480:string)
              n457 = GPIB Write(0:w470, 1:w480) -> (6:w469:errorcluster)  [unwired: 3 in, 1 out]
            }
            frame #1 {
              n458 = stacked-sequence {
                tunnel: w873 -> [w876 _ _ _ _ _ _ _ _ _ _ _ _ _ _ _ _ _ _ _ _ _ _ _ _ _]
                tunnel: [w876 _ _ _ _ _ _ _ _ _ _ _ _ _ _ _ _ _ _ _ _ _ _ _ _ _] -> w859
                frame #0 {
                  # "check if oscillator on \nlock-in (address 1)\nis to be measured"
                  n459 = property on="Current is:" class="RadioBtnsControl (strict)"() -> ("Value"=w879:T1)  [unwired: 2 in, 2 out]
                  n460 = property on="array for data" class="Arr (strict)"() -> ("Value"=w878:dbl[])  [unwired: 2 in, 2 out]
                  n461 = Equal?(x=w879, y=1) -> (x = y?=w880:bool)
                  n462 = case shown="False" w880 {
                    tunnel: w878 -> [w882 w890]
                    tunnel: [w882 w889] -> w877
                    frame False {
                      # "we are not measuring oscillator from\nlock-in (address 1)"
                    }
                    frame True {
                      w886 = "1"
                      # "we are  measuring oscillator"
                      n463 = GPIB Write(0:w886, 1:"SLVL?") -> (6:w887:errorcluster)  [unwired: 3 in, 1 out]
                      n464 = GPIB Read(0:w886, 1:3200, 3:w887) -> (5:w884:string)  [unwired: 2 in, 2 out]
                      n465 = Fract/Exp String To Number(string=w884) -> (number=w883:dbl)  [unwired: 3 in, 1 out]
                      n466 = Build Array (concatenate)(w890, w883) -> (w889:dbl[])
                    }
                  }
                  n467 = property on="array for data" class="Arr (strict)"("Value"=w877) -> ()  [unwired: 2 in, 2 out]
                }
                frame #1 {
                  # "check if in-phase\nsignal on lock-in \n(address 1) is to\nbe measured"
                  n468 = property on="array for data" class="Arr (strict)"() -> ("Value"=w893:dbl[])  [unwired: 2 in, 2 out]
                  n469 = property on="Addr 1 lock-in" class="Bool (strict)"() -> ("Value"=w891:bool)  [unwired: 2 in, 2 out]
                  n470 = case shown="True" w891 {
                    tunnel: w893 -> [w894 w902]
                    tunnel: [w894 w901] -> w892
                    frame False {
                      # "we are not measuring in phase signal on lock-in (address 1)"
                    }
                    frame True {
                      w899 = "1"
                      # "we are  measuring lock-in (address 1), in phase"
                      n471 = GPIB Write(0:w899, 1:"OUTP?1") -> (6:w900:errorcluster)  [unwired: 3 in, 1 out]
                      n472 = GPIB Read(0:w899, 1:3200, 3:w900) -> (5:w897:string)  [unwired: 2 in, 2 out]
                      n473 = Fract/Exp String To Number(string=w897) -> (number=w896:dbl)  [unwired: 3 in, 1 out]
                      n474 = Build Array (concatenate)(w902, w896) -> (w901:dbl[])
                    }
                  }
                  n475 = property on="array for data" class="Arr (strict)"("Value"=w892) -> ()  [unwired: 2 in, 2 out]
                }
                frame #2 {
                  # "check if out-of-phase\nsignal on lock-in \n(address 1) is to\nbe measured"
                  n476 = property on="Addr 1 lock-in oop" class="Bool (strict)"() -> ("Value"=w903:bool)  [unwired: 2 in, 2 out]
                  n477 = property on="array for data" class="Arr (strict)"() -> ("Value"=w905:dbl[])  [unwired: 2 in, 2 out]
                  n478 = case shown="True" w903 {
                    tunnel: w905 -> [w906 w914]
                    tunnel: [w906 w913] -> w904
                    frame False {
                      # "we are not measuring out-of-phase signal on lock-in (address 1)"
                    }
                    frame True {
                      w911 = "1"
                      # "we are  measuring lock-in (address 1), out-of-phase signal"
                      n479 = GPIB Write(0:w911, 1:"OUTP?2") -> (6:w912:errorcluster)  [unwired: 3 in, 1 out]
                      n480 = GPIB Read(0:w911, 1:3200, 3:w912) -> (5:w909:string)  [unwired: 2 in, 2 out]
                      n481 = Fract/Exp String To Number(string=w909) -> (number=w908:dbl)  [unwired: 3 in, 1 out]
                      n482 = Build Array (concatenate)(w914, w908) -> (w913:dbl[])
                    }
                  }
                  n483 = property on="array for data" class="Arr (strict)"("Value"=w904) -> ()  [unwired: 2 in, 2 out]
                }
                frame #3 {
                  # "check if in-phase\nsignal on lock-in \n(address 2) is to\nbe measured"
                  n484 = property on="Addr 2 lock-in" class="Bool (strict)"() -> ("Value"=w915:bool)  [unwired: 2 in, 2 out]
                  n485 = property on="array for data" class="Arr (strict)"() -> ("Value"=w917:dbl[])  [unwired: 2 in, 2 out]
                  n486 = case shown="False" w915 {
                    tunnel: w917 -> [w918 w926]
                    tunnel: [w918 w925] -> w916
                    frame False {
                      # "we are not measuring in phase signal on lock-in (address 2)"
                    }
                    frame True {
                      w923 = "2"
                      # "we are  measuring lock-in (address 2), in phase"
                      n487 = GPIB Write(0:w923, 1:"OUTP?1") -> (6:w924:errorcluster)  [unwired: 3 in, 1 out]
                      n488 = GPIB Read(0:w923, 1:3200, 3:w924) -> (5:w921:string)  [unwired: 2 in, 2 out]
                      n489 = Fract/Exp String To Number(string=w921) -> (number=w920:dbl)  [unwired: 3 in, 1 out]
                      n490 = Build Array (concatenate)(w926, w920) -> (w925:dbl[])
                    }
                  }
                  n491 = property on="array for data" class="Arr (strict)"("Value"=w916) -> ()  [unwired: 2 in, 2 out]
                }
                frame #4 {
                  # "check if out-of-phase\nsignal on lock-in \n(address 2) is to\nbe measured"
                  n492 = property on="Addr 2 lock-in oop" class="Bool (strict)"() -> ("Value"=w927:bool)  [unwired: 2 in, 2 out]
                  n493 = property on="array for data" class="Arr (strict)"() -> ("Value"=w929:dbl[])  [unwired: 2 in, 2 out]
                  n494 = case shown="False" w927 {
                    tunnel: w929 -> [w930 w938]
                    tunnel: [w930 w937] -> w928
                    tunnel: w927 -> [_ _]
                    frame False {
                      # "we are not measuring out-of-phase signal on lock-in (address 2)"
                    }
                    frame True {
                      w935 = "2"
                      # "we are  measuring lock-in (address 2), out-of-phase"
                      n495 = GPIB Write(0:w935, 1:"OUTP?2") -> (6:w936:errorcluster)  [unwired: 3 in, 1 out]
                      n496 = GPIB Read(0:w935, 1:3200, 3:w936) -> (5:w933:string)  [unwired: 2 in, 2 out]
                      n497 = Fract/Exp String To Number(string=w933) -> (number=w932:dbl)  [unwired: 3 in, 1 out]
                      n498 = Build Array (concatenate)(w938, w932) -> (w937:dbl[])
                    }
                  }
                  n499 = property on="array for data" class="Arr (strict)"("Value"=w928) -> ()  [unwired: 2 in, 2 out]
                }
                frame #5 {
                  # "check if in-phase\nsignal on lock-in \n(address 3) is to\nbe measured"
                  n500 = property on="Addr 3 lock-in" class="Bool (strict)"() -> ("Value"=w939:bool)  [unwired: 2 in, 2 out]
                  n501 = property on="array for data" class="Arr (strict)"() -> ("Value"=w941:dbl[])  [unwired: 2 in, 2 out]
                  n502 = case shown="True" w939 {
                    tunnel: w941 -> [w942 w950]
                    tunnel: [w942 w949] -> w940
                    frame False {
                      # "we are not measuring in phase signal on lock-in (address 3)"
                    }
                    frame True {
                      w947 = "3"
                      # "we are  measuring lock-in (address 3), in phase"
                      n503 = GPIB Write(0:w947, 1:"OUTP?1") -> (6:w948:errorcluster)  [unwired: 3 in, 1 out]
                      n504 = GPIB Read(0:w947, 1:3200, 3:w948) -> (5:w945:string)  [unwired: 2 in, 2 out]
                      n505 = Fract/Exp String To Number(string=w945) -> (number=w944:dbl)  [unwired: 3 in, 1 out]
                      n506 = Build Array (concatenate)(w950, w944) -> (w949:dbl[])
                    }
                  }
                  n507 = property on="array for data" class="Arr (strict)"("Value"=w940) -> ()  [unwired: 2 in, 2 out]
                }
                frame #6 {
                  # "check if out-of-phase\nsignal on lock-in \n(address 3) is to\nbe measured"
                  n508 = property on="Addr 3 lock-in oop" class="Bool (strict)"() -> ("Value"=w951:bool)  [unwired: 2 in, 2 out]
                  n509 = property on="array for data" class="Arr (strict)"() -> ("Value"=w953:dbl[])  [unwired: 2 in, 2 out]
                  n510 = case shown="True" w951 {
                    tunnel: w953 -> [w954 w962]
                    tunnel: [w954 w961] -> w952
                    frame False {
                      # "we are not measuring out-of-phase signal on lock-in (address 3)"
                    }
                    frame True {
                      w959 = "3"
                      # "we are  measuring lock-in (address 3), out-of-phase"
                      n511 = GPIB Write(0:w959, 1:"OUTP?2") -> (6:w960:errorcluster)  [unwired: 3 in, 1 out]
                      n512 = GPIB Read(0:w959, 1:3200, 3:w960) -> (5:w957:string)  [unwired: 2 in, 2 out]
                      n513 = Fract/Exp String To Number(string=w957) -> (number=w956:dbl)  [unwired: 3 in, 1 out]
                      n514 = Build Array (concatenate)(w962, w956) -> (w961:dbl[])
                    }
                  }
                  n515 = property on="array for data" class="Arr (strict)"("Value"=w952) -> ()  [unwired: 2 in, 2 out]
                }
                frame #7 {
                  # "check if in-phase\nsignal on lock-in \n(address 4) is to\nbe measured"
                  n516 = property on="Addr 4 lock-in" class="Bool (strict)"() -> ("Value"=w963:bool)  [unwired: 2 in, 2 out]
                  n517 = property on="array for data" class="Arr (strict)"() -> ("Value"=w965:dbl[])  [unwired: 2 in, 2 out]
                  n518 = case shown="True" w963 {
                    tunnel: w965 -> [w966 w974]
                    tunnel: [w966 w973] -> w964
                    frame False {
                      # "we are not measuring in phase signal on lock-in (address 4)"
                    }
                    frame True {
                      w971 = "4"
                      # "we are  measuring lock-in (address 4), in phase"
                      n519 = GPIB Write(0:w971, 1:"OUTP?1") -> (6:w972:errorcluster)  [unwired: 3 in, 1 out]
                      n520 = GPIB Read(0:w971, 1:3200, 3:w972) -> (5:w969:string)  [unwired: 2 in, 2 out]
                      n521 = Fract/Exp String To Number(string=w969) -> (number=w968:dbl)  [unwired: 3 in, 1 out]
                      n522 = Build Array (concatenate)(w974, w968) -> (w973:dbl[])
                    }
                  }
                  n523 = property on="array for data" class="Arr (strict)"("Value"=w964) -> ()  [unwired: 2 in, 2 out]
                }
                frame #8 {
                  # "check if out-of-phase\nsignal on lock-in \n(address 4) is to\nbe measured"
                  n524 = property on="Addr 4 lock-in oop" class="Bool (strict)"() -> ("Value"=w975:bool)  [unwired: 2 in, 2 out]
                  n525 = property on="array for data" class="Arr (strict)"() -> ("Value"=w977:dbl[])  [unwired: 2 in, 2 out]
                  n526 = case shown="True" w975 {
                    tunnel: w977 -> [w978 w986]
                    tunnel: [w978 w985] -> w976
                    frame False {
                      # "we are not measuring out-of-phase signal on lock-in (address 4)"
                    }
                    frame True {
                      w983 = "4"
                      # "we are  measuring lock-in (address 4), out-of-phase"
                      n527 = GPIB Write(0:w983, 1:"OUTP?2") -> (6:w984:errorcluster)  [unwired: 3 in, 1 out]
                      n528 = GPIB Read(0:w983, 1:3200, 3:w984) -> (5:w981:string)  [unwired: 2 in, 2 out]
                      n529 = Fract/Exp String To Number(string=w981) -> (number=w980:dbl)  [unwired: 3 in, 1 out]
                      n530 = Build Array (concatenate)(w986, w980) -> (w985:dbl[])
                    }
                  }
                  n531 = property on="array for data" class="Arr (strict)"("Value"=w976) -> ()  [unwired: 2 in, 2 out]
                }
                frame #9 {
                  # "check if in-phase\nsignal on lock-in \n(address 5) is to\nbe measured"
                  n532 = property on="Addr 5 lock-in" class="Bool (strict)"() -> ("Value"=w987:bool)  [unwired: 2 in, 2 out]
                  n533 = property on="array for data" class="Arr (strict)"() -> ("Value"=w989:dbl[])  [unwired: 2 in, 2 out]
                  n534 = case shown="False" w987 {
                    tunnel: w989 -> [w990 w998]
                    tunnel: [w990 w997] -> w988
                    frame False {
                      # "we are not measuring in phase signal on lock-in (address 5)"
                    }
                    frame True {
                      w995 = "5"
                      # "we are  measuring lock-in (address 5), in phase"
                      n535 = GPIB Write(0:w995, 1:"OUTP?1") -> (6:w996:errorcluster)  [unwired: 3 in, 1 out]
                      n536 = GPIB Read(0:w995, 1:3200, 3:w996) -> (5:w993:string)  [unwired: 2 in, 2 out]
                      n537 = Fract/Exp String To Number(string=w993) -> (number=w992:dbl)  [unwired: 3 in, 1 out]
                      n538 = Build Array (concatenate)(w998, w992) -> (w997:dbl[])
                    }
                  }
                  n539 = property on="array for data" class="Arr (strict)"("Value"=w988) -> ()  [unwired: 2 in, 2 out]
                }
                frame #10 {
                  # "check if out-of-phase\nsignal on lock-in \n(address 5) is to\nbe measured"
                  n540 = property on="Addr 5 lock-in oop" class="Bool (strict)"() -> ("Value"=w999:bool)  [unwired: 2 in, 2 out]
                  n541 = property on="array for data" class="Arr (strict)"() -> ("Value"=w1001:dbl[])  [unwired: 2 in, 2 out]
                  n542 = case shown="False" w999 {
                    tunnel: w1001 -> [w1002 w1010]
                    tunnel: [w1002 w1009] -> w1000
                    frame False {
                      # "we are not measuring out-of-phase signal on lock-in (address 5)"
                    }
                    frame True {
                      w1007 = "5"
                      # "we are  measuring lock-in (address 5), out-of-phase"
                      n543 = GPIB Write(0:w1007, 1:"OUTP?2") -> (6:w1008:errorcluster)  [unwired: 3 in, 1 out]
                      n544 = GPIB Read(0:w1007, 1:3200, 3:w1008) -> (5:w1005:string)  [unwired: 2 in, 2 out]
                      n545 = Fract/Exp String To Number(string=w1005) -> (number=w1004:dbl)  [unwired: 3 in, 1 out]
                      n546 = Build Array (concatenate)(w1010, w1004) -> (w1009:dbl[])
                    }
                  }
                  n547 = property on="array for data" class="Arr (strict)"("Value"=w1000) -> ()  [unwired: 2 in, 2 out]
                }
                frame #11 {
                  # "check if voltage on \nmain Keithley 2400 \n(addr. 12) is to\nbe measured"
                  n548 = property on="Voltage (Vk1)" class="Bool (strict)"() -> ("Value"=w1011:bool)  [unwired: 2 in, 2 out]
                  n549 = property on="array for data" class="Arr (strict)"() -> ("Value"=w1013:dbl[])  [unwired: 2 in, 2 out]
                  n550 = case shown="False" w1011 {
                    tunnel: w1013 -> [w1014 w1024]
                    tunnel: [w1014 w1023] -> w1012
                    frame False {
                      # "we aren't measuring voltage \non main Keithley 2400 (addr. 12)"
                    }
                    frame True {
                      w1021 = "12"
                      # "we are measuring voltage \non main Keithley 2400 (addr. 12)"
                      n551 = GPIB Write(0:w1021, 1:":READ?") -> (6:w1022:errorcluster)  [unwired: 3 in, 1 out]
                      n552 = GPIB Read(0:w1021, 1:3200, 3:w1022) -> (5:w1017:string)  [unwired: 2 in, 2 out]
                      n553 = String Subset(string=w1017, length (rest)=13) -> (substring=w1016:string)  [unwired: 1 in]
                      n554 = Fract/Exp String To Number(string=w1016) -> (number=w1019:dbl)  [unwired: 3 in, 1 out]
                      n555 = Build Array (concatenate)(w1024, w1019) -> (w1023:dbl[])
                    }
                  }
                  n556 = property on="array for data" class="Arr (strict)"("Value"=w1012) -> ()  [unwired: 2 in, 2 out]
                }
                frame #12 {
                  # "check if  current on \nmain Keithley 2400 \n(addr. 12) is to\nbe measured"
                  n557 = property on="Current (Ik1)" class="Bool (strict)"() -> ("Value"=w1025:bool)  [unwired: 2 in, 2 out]
                  n558 = property on="array for data" class="Arr (strict)"() -> ("Value"=w1027:dbl[])  [unwired: 2 in, 2 out]
                  n559 = case shown="True" w1025 {
                    tunnel: w1027 -> [w1028 w1039]
                    tunnel: [w1028 w1038] -> w1026
                    frame False {
                      # "we aren't measuring current \non main Keithley 2400 (addr. 12)"
                    }
                    frame True {
                      w1036 = "12"
                      # "we are measuring current\non main Keithley 2400 (addr. 12)"
                      n560 = GPIB Write(0:w1036, 1:":READ?") -> (6:w1037:errorcluster)  [unwired: 3 in, 1 out]
                      n561 = GPIB Read(0:w1036, 1:3200, 3:w1037) -> (5:w1032:string)  [unwired: 2 in, 2 out]
                      n562 = String Subset(string=w1032, offset (0)=14, length (rest)=13) -> (substring=w1031:string)
                      n563 = Fract/Exp String To Number(string=w1031) -> (number=w1034:dbl)  [unwired: 3 in, 1 out]
                      n564 = Build Array (concatenate)(w1039, w1034) -> (w1038:dbl[])
                    }
                  }
                  n565 = property on="array for data" class="Arr (strict)"("Value"=w1026) -> ()  [unwired: 2 in, 2 out]
                }
                frame #13 {
                  # "check if voltage on \nadd. Keithley 2400 \n(addr. 13) is to\nbe measured"
                  n566 = property on="Voltage (Vk2)" class="Bool (strict)"() -> ("Value"=w1040:bool)  [unwired: 2 in, 2 out]
                  n567 = property on="array for data" class="Arr (strict)"() -> ("Value"=w1042:dbl[])  [unwired: 2 in, 2 out]
                  n568 = case shown="True" w1040 {
                    tunnel: w1042 -> [w1043 w1053]
                    tunnel: [w1043 w1052] -> w1041
                    frame False {
                      # "we aren't measuring voltage \non additional Keithley 2400 (addr. 13)"
                    }
                    frame True {
                      w1050 = "13"
                      # "we are measuring voltage \non additional Keithley 2400 (addr. 13)"
                      n569 = GPIB Write(0:w1050, 1:":READ?") -> (6:w1051:errorcluster)  [unwired: 3 in, 1 out]
                      n570 = GPIB Read(0:w1050, 1:3200, 3:w1051) -> (5:w1046:string)  [unwired: 2 in, 2 out]
                      n571 = String Subset(string=w1046, length (rest)=13) -> (substring=w1045:string)  [unwired: 1 in]
                      n572 = Fract/Exp String To Number(string=w1045) -> (number=w1048:dbl)  [unwired: 3 in, 1 out]
                      n573 = Build Array (concatenate)(w1053, w1048) -> (w1052:dbl[])
                    }
                  }
                  n574 = property on="array for data" class="Arr (strict)"("Value"=w1041) -> ()  [unwired: 2 in, 2 out]
                }
                frame #14 {
                  # "check if  current on \nadd. Keithley 2400 \n(addr. 13) is to\nbe measured"
                  n575 = property on="Current (Ik2)" class="Bool (strict)"() -> ("Value"=w1054:bool)  [unwired: 2 in, 2 out]
                  n576 = property on="array for data" class="Arr (strict)"() -> ("Value"=w1056:dbl[])  [unwired: 2 in, 2 out]
                  n577 = case shown="True" w1054 {
                    tunnel: w1056 -> [w1057 w1068]
                    tunnel: [w1057 w1067] -> w1055
                    frame False {
                      # "we aren't measuring current \non additional Keithley 2400 (addr. 13)"
                    }
                    frame True {
                      w1065 = "13"
                      # "we are measuring current\non additional Keithley 2400 (addr. 13)"
                      n578 = GPIB Write(0:w1065, 1:":READ?") -> (6:w1066:errorcluster)  [unwired: 3 in, 1 out]
                      n579 = GPIB Read(0:w1065, 1:3200, 3:w1066) -> (5:w1061:string)  [unwired: 2 in, 2 out]
                      n580 = String Subset(string=w1061, offset (0)=14, length (rest)=13) -> (substring=w1060:string)
                      n581 = Fract/Exp String To Number(string=w1060) -> (number=w1063:dbl)  [unwired: 3 in, 1 out]
                      n582 = Build Array (concatenate)(w1068, w1063) -> (w1067:dbl[])
                    }
                  }
                  n583 = property on="array for data" class="Arr (strict)"("Value"=w1055) -> ()  [unwired: 2 in, 2 out]
                }
                frame #15 {
                  # "check if voltage on \nadd. Keithley 2400 \n(addr. 14) is to\nbe measured"
                  n584 = property on="Voltage (Vk3)" class="Bool (strict)"() -> ("Value"=w1069:bool)  [unwired: 2 in, 2 out]
                  n585 = property on="array for data" class="Arr (strict)"() -> ("Value"=w1071:dbl[])  [unwired: 2 in, 2 out]
                  n586 = case shown="False" w1069 {
                    tunnel: w1071 -> [w1072 w1082]
                    tunnel: [w1072 w1081] -> w1070
                    frame False {
                      # "we aren't measuring voltage \non additional Keithley 2400 (addr. 14)"
                    }
                    frame True {
                      w1079 = "14"
                      # "we are measuring voltage \non additional Keithley 2400 (addr. 14)"
                      n587 = GPIB Write(0:w1079, 1:":READ?") -> (6:w1080:errorcluster)  [unwired: 3 in, 1 out]
                      n588 = GPIB Read(0:w1079, 1:3200, 3:w1080) -> (5:w1075:string)  [unwired: 2 in, 2 out]
                      n589 = String Subset(string=w1075, length (rest)=13) -> (substring=w1074:string)  [unwired: 1 in]
                      n590 = Fract/Exp String To Number(string=w1074) -> (number=w1077:dbl)  [unwired: 3 in, 1 out]
                      n591 = Build Array (concatenate)(w1082, w1077) -> (w1081:dbl[])
                    }
                  }
                  n592 = property on="array for data" class="Arr (strict)"("Value"=w1070) -> ()  [unwired: 2 in, 2 out]
                }
                frame #16 {
                  # "check if  current on \nadd. Keithley 2400 \n(addr. 14) is to\nbe measured"
                  n593 = property on="Current (Ik3)" class="Bool (strict)"() -> ("Value"=w1083:bool)  [unwired: 2 in, 2 out]
                  n594 = property on="array for data" class="Arr (strict)"() -> ("Value"=w1085:dbl[])  [unwired: 2 in, 2 out]
                  n595 = case shown="True" w1083 {
                    tunnel: w1085 -> [w1086 w1097]
                    tunnel: [w1086 w1096] -> w1084
                    frame False {
                      # "we aren't measuring current \non additional Keithley 2400 (addr. 14)"
                    }
                    frame True {
                      w1094 = "14"
                      # "we are measuring current\non additional Keithley 2400 (addr. 14)"
                      n596 = GPIB Write(0:w1094, 1:":READ?") -> (6:w1095:errorcluster)  [unwired: 3 in, 1 out]
                      n597 = GPIB Read(0:w1094, 1:3200, 3:w1095) -> (5:w1090:string)  [unwired: 2 in, 2 out]
                      n598 = String Subset(string=w1090, offset (0)=14, length (rest)=13) -> (substring=w1089:string)
                      n599 = Fract/Exp String To Number(string=w1089) -> (number=w1092:dbl)  [unwired: 3 in, 1 out]
                      n600 = Build Array (concatenate)(w1097, w1092) -> (w1096:dbl[])
                    }
                  }
                  n601 = property on="array for data" class="Arr (strict)"("Value"=w1084) -> ()  [unwired: 2 in, 2 out]
                }
                frame #17 {
                  # "check if 1st channel\non Keithley 2182 \n(addr. 15) is to\nbe measured"
                  n602 = property on="Channel 1 (Vnano1)" class="Bool (strict)"() -> ("Value"=w1098:bool)  [unwired: 2 in, 2 out]
                  n603 = property on="array for data" class="Arr (strict)"() -> ("Value"=w1100:dbl[])  [unwired: 2 in, 2 out]
                  n604 = case shown="True" w1098 {
                    tunnel: w1100 -> [w1101 w1109]
                    tunnel: [w1101 w1108] -> w1099
                    frame False {
                      # "we are not measuring 1st channel\non Keithley 2182 (addr. 15)"
                    }
                    frame True {
                      w1106 = "15"
                      # "we are measuring 1st channel\non Keithley 2182 (addr. 15)"
                      n605 = GPIB Write(0:w1106, 1:":SENSe:DATA:FRES?") -> (6:w1107:errorcluster)  [unwired: 3 in, 1 out]
                      n606 = GPIB Read(0:w1106, 1:200, 3:w1107) -> (5:w1102:string)  [unwired: 2 in, 2 out]
                      n607 = Fract/Exp String To Number(string=w1102) -> (number=w1104:dbl)  [unwired: 3 in, 1 out]
                      n608 = Build Array (concatenate)(w1109, w1104) -> (w1108:dbl[])
                    }
                  }
                  n609 = property on="array for data" class="Arr (strict)"("Value"=w1099) -> ()  [unwired: 2 in, 2 out]
                }
                frame #18 {
                  # "check if 2nd channel\non Keithley 2182 \n(addr. 15) is to\nbe measured"
                  n610 = property on="Channel 2 (Vnano1b)" class="Bool (strict)"() -> ("Value"=w1110:bool)  [unwired: 2 in, 2 out]
                  n611 = property on="array for data" class="Arr (strict)"() -> ("Value"=w1112:dbl[])  [unwired: 2 in, 2 out]
                  n612 = case shown="False" w1110 {
                    tunnel: w1112 -> [w1113 w1125]
                    tunnel: [w1113 w1124] -> w1111
                    frame False {
                      # "we are not measuring 1st channel\non Keithley 2182 (addr. 15)"
                    }
                    frame True {
                      w1116 = "15"
                      # "switching to channel 2 and then\nback to channel 1"
                      # "we are measuring 2nd channel\non Keithley 2182 (addr. 15)"
                      n613 = GPIB Write(0:w1116, 1:":SENSe:CHAN 2") -> (6:w1117:errorcluster)  [unwired: 3 in, 1 out]
                      n614 = GPIB Write(0:w1116, 1:":SENSe:DATA:FRES?", 3:w1117) -> (6:w1123:errorcluster)  [unwired: 2 in, 1 out]
                      n615 = GPIB Read(0:w1116, 1:200, 3:w1123) -> (5:w1119:string, 7:w1115:errorcluster)  [unwired: 2 in, 1 out]
                      n616 = GPIB Write(0:w1116, 1:":SENSe:CHAN 1", 3:w1115) -> ()  [unwired: 2 in, 2 out]
                      n617 = Fract/Exp String To Number(string=w1119) -> (number=w1121:dbl)  [unwired: 3 in, 1 out]
                      n618 = Build Array (concatenate)(w1125, w1121) -> (w1124:dbl[])
                    }
                  }
                  n619 = property on="array for data" class="Arr (strict)"("Value"=w1111) -> ()  [unwired: 2 in, 2 out]
                }
                frame #19 {
                  # "check if 1st channel\non Keithley 2182 \n(addr. 16) is to\nbe measured"
                  n620 = property on="Channel 1 (Vnano2)" class="Bool (strict)"() -> ("Value"=w1126:bool)  [unwired: 2 in, 2 out]
                  n621 = property on="array for data" class="Arr (strict)"() -> ("Value"=w1128:dbl[])  [unwired: 2 in, 2 out]
                  n622 = case shown="True" w1126 {
                    tunnel: w1128 -> [w1129 w1137]
                    tunnel: [w1129 w1136] -> w1127
                    frame False {
                      # "we are not measuring 1st channel\non Keithley 2182 (addr. 16)"
                    }
                    frame True {
                      w1134 = "16"
                      # "we are measuring 1st channel\non Keithley 2182 (addr. 16)"
                      n623 = GPIB Write(0:w1134, 1:":SENSe:DATA:FRES?") -> (6:w1135:errorcluster)  [unwired: 3 in, 1 out]
                      n624 = GPIB Read(0:w1134, 1:200, 3:w1135) -> (5:w1130:string)  [unwired: 2 in, 2 out]
                      n625 = Fract/Exp String To Number(string=w1130) -> (number=w1132:dbl)  [unwired: 3 in, 1 out]
                      n626 = Build Array (concatenate)(w1137, w1132) -> (w1136:dbl[])
                    }
                  }
                  n627 = property on="array for data" class="Arr (strict)"("Value"=w1127) -> ()  [unwired: 2 in, 2 out]
                }
                frame #20 {
                  # "check if 2nd channel\non Keithley 2182 \n(addr. 16) is to\nbe measured"
                  n628 = property on="Channel 2 (Vnano2b)" class="Bool (strict)"() -> ("Value"=w1138:bool)  [unwired: 2 in, 2 out]
                  n629 = property on="array for data" class="Arr (strict)"() -> ("Value"=w1140:dbl[])  [unwired: 2 in, 2 out]
                  n630 = case shown="True" w1138 {
                    tunnel: w1140 -> [w1141 w1153]
                    tunnel: [w1141 w1152] -> w1139
                    frame False {
                      # "we are not measuring 1st channel\non Keithley 2182 (addr. 16)"
                    }
                    frame True {
                      w1144 = "16"
                      # "switching to channel 2 and then\nback to channel 1"
                      # "we are measuring 2nd channel\non Keithley 2182 (addr. 16)"
                      n631 = GPIB Write(0:w1144, 1:":SENSe:CHAN 2") -> (6:w1145:errorcluster)  [unwired: 3 in, 1 out]
                      n632 = GPIB Write(0:w1144, 1:":SENSe:DATA:FRES?", 3:w1145) -> (6:w1151:errorcluster)  [unwired: 2 in, 1 out]
                      n633 = GPIB Read(0:w1144, 1:200, 3:w1151) -> (5:w1147:string, 7:w1143:errorcluster)  [unwired: 2 in, 1 out]
                      n634 = GPIB Write(0:w1144, 1:":SENSe:CHAN 1", 3:w1143) -> ()  [unwired: 2 in, 2 out]
                      n635 = Fract/Exp String To Number(string=w1147) -> (number=w1149:dbl)  [unwired: 3 in, 1 out]
                      n636 = Build Array (concatenate)(w1153, w1149) -> (w1152:dbl[])
                    }
                  }
                  n637 = property on="array for data" class="Arr (strict)"("Value"=w1139) -> ()  [unwired: 2 in, 2 out]
                }
                frame #21 {
                  # "check if 1st channel\non Keithley 2182 \n(addr. 17) is to\nbe measured"
                  n638 = property on="Channel 1 (Vnano3)" class="Bool (strict)"() -> ("Value"=w1154:bool)  [unwired: 2 in, 2 out]
                  n639 = property on="array for data" class="Arr (strict)"() -> ("Value"=w1156:dbl[])  [unwired: 2 in, 2 out]
                  n640 = case shown="True" w1154 {
                    tunnel: w1156 -> [w1157 w1165]
                    tunnel: [w1157 w1164] -> w1155
                    frame False {
                      # "we are not measuring 1st channel\non Keithley 2182 (addr. 17)"
                    }
                    frame True {
                      w1162 = "17"
                      # "we are measuring 1st channel\non Keithley 2182 (addr. 17)"
                      n641 = GPIB Write(0:w1162, 1:":SENSe:DATA:FRES?") -> (6:w1163:errorcluster)  [unwired: 3 in, 1 out]
                      n642 = GPIB Read(0:w1162, 1:200, 3:w1163) -> (5:w1158:string)  [unwired: 2 in, 2 out]
                      n643 = Fract/Exp String To Number(string=w1158) -> (number=w1160:dbl)  [unwired: 3 in, 1 out]
                      n644 = Build Array (concatenate)(w1165, w1160) -> (w1164:dbl[])
                    }
                  }
                  n645 = property on="array for data" class="Arr (strict)"("Value"=w1155) -> ()  [unwired: 2 in, 2 out]
                }
                frame #22 {
                  # "check if 2nd channel\non Keithley 2182 \n(addr. 17) is to\nbe measured"
                  n646 = property on="Channel 2 (Vnano3b)" class="Bool (strict)"() -> ("Value"=w1166:bool)  [unwired: 2 in, 2 out]
                  n647 = property on="array for data" class="Arr (strict)"() -> ("Value"=w1168:dbl[])  [unwired: 2 in, 2 out]
                  n648 = case shown="True" w1166 {
                    tunnel: w1168 -> [w1169 w1181]
                    tunnel: [w1169 w1180] -> w1167
                    frame False {
                      # "we are not measuring 1st channel\non Keithley 2182 (addr. 17)"
                    }
                    frame True {
                      w1172 = "17"
                      # "switching to channel 2 and then\nback to channel 1"
                      # "we are measuring 2nd channel\non Keithley 2182 (addr. 17)"
                      n649 = GPIB Write(0:w1172, 1:":SENSe:CHAN 2") -> (6:w1173:errorcluster)  [unwired: 3 in, 1 out]
                      n650 = GPIB Write(0:w1172, 1:":SENSe:DATA:FRES?", 3:w1173) -> (6:w1179:errorcluster)  [unwired: 2 in, 1 out]
                      n651 = GPIB Read(0:w1172, 1:200, 3:w1179) -> (5:w1175:string, 7:w1171:errorcluster)  [unwired: 2 in, 1 out]
                      n652 = GPIB Write(0:w1172, 1:":SENSe:CHAN 1", 3:w1171) -> ()  [unwired: 2 in, 2 out]
                      n653 = Fract/Exp String To Number(string=w1175) -> (number=w1177:dbl)  [unwired: 3 in, 1 out]
                      n654 = Build Array (concatenate)(w1181, w1177) -> (w1180:dbl[])
                    }
                  }
                  n655 = property on="array for data" class="Arr (strict)"("Value"=w1167) -> ()  [unwired: 2 in, 2 out]
                }
                frame #23 {
                  # "check if 1st \nthermometer on \nOxford ITC \n(address 24) \nis measured"
                  n656 = property on="Thermometer 1 (T1)" class="Bool (strict)"() -> ("Value"=w1182:bool)  [unwired: 2 in, 2 out]
                  n657 = property on="array for data" class="Arr (strict)"() -> ("Value"=w1184:dbl[])  [unwired: 2 in, 2 out]
                  n658 = case shown="True" w1182 {
                    tunnel: w1184 -> [w1185 w1194]
                    tunnel: [w1185 w1193] -> w1183
                    frame False {
                      # "we are not measuring temperature on\nthermometer 1 (addr. 24)"
                    }
                    frame True {
                      w1186 = 1
                      w1191 = "24"
                      # "we are measuring temperature,\nthermometer 1 (addr. 24)"
                      n659 = GPIB Write(0:w1191, 1:"R 1", 2:w1186) -> (6:w1192:errorcluster)  [unwired: 2 in, 1 out]
                      n660 = GPIB Read(0:w1191, 1:200, 2:w1186, 3:w1192) -> (5:w1187:string)  [unwired: 1 in, 2 out]
                      n661 = Fract/Exp String To Number(string=w1187, offset=w1186) -> (number=w1189:dbl)  [unwired: 2 in, 1 out]
                      n662 = Build Array (concatenate)(w1194, w1189) -> (w1193:dbl[])
                    }
                  }
                  n663 = property on="array for data" class="Arr (strict)"("Value"=w1183) -> ()  [unwired: 2 in, 2 out]
                }
                frame #24 {
                  # "check if 1st \nthermometer on \nOxford ITC \n(address 24) \nis measured"
                  n664 = property on="Magnetic Field (B)" class="Bool (strict)"() -> ("Value"=w1195:bool)  [unwired: 2 in, 2 out]
                  n665 = property on="array for data" class="Arr (strict)"() -> ("Value"=w1197:dbl[])  [unwired: 2 in, 2 out]
                  n666 = case shown="True" w1195 {
                    tunnel: w1197 -> [w1198 w1207]
                    tunnel: [w1198 w1206] -> w1196
                    frame False {
                      # "we are not measuringmagnetic field (addr. 25)"
                    }
                    frame True {
                      w1199 = 1
                      w1204 = "25"
                      # "we are measuring magnetic field  (addr. 25)"
                      n667 = GPIB Write(0:w1204, 1:"R 8", 2:w1199) -> (6:w1205:errorcluster)  [unwired: 2 in, 1 out]
                      n668 = GPIB Read(0:w1204, 1:200, 2:w1199, 3:w1205) -> (5:w1200:string)  [unwired: 1 in, 2 out]
                      n669 = Fract/Exp String To Number(string=w1200, offset=w1199) -> (number=w1202:dbl)  [unwired: 2 in, 1 out]
                      n670 = Build Array (concatenate)(w1207, w1202) -> (w1206:dbl[])
                    }
                  }
                  n671 = property on="array for data" class="Arr (strict)"("Value"=w1196) -> ()  [unwired: 2 in, 2 out]
                }
                frame #25 {
                  # "check if capacitance\nand loss (address 28)\nare measured"
                  n672 = property on="Capacitance (C) and Loss (L)" class="Bool (strict)"() -> ("Value"=w1208:bool)  [unwired: 2 in, 2 out]
                  n673 = property on="array for data" class="Arr (strict)"() -> ("Value"=w1210:dbl[])  [unwired: 2 in, 2 out]
                  n674 = case shown="True" w1208 {
                    tunnel: w1210 -> [w1211 w1217]
                    tunnel: [w1211 w1213] -> w1209
                    frame False {
                      # "we are not measuringmagnetic capacitance (addr. 28)"
                    }
                    frame True {
                      # "we are measuring capacitance and loss  (addr. 28)"
                      n675 = stacked-sequence {
                        seq-local: [w1219 _ _] -> [_ _ w1242]
                        tunnel: [_ _ w1236] -> w1212
                        tunnel: [_ _ w1237] -> w1215
                        tunnel: "28" ("data") -> [w1218 w1222 w1231]
                        frame #0 {
                          n676 = GPIB Write(0:w1218, 1:"SINGLE" ("data"), 2:i16 0 ("mode (0)")) -> (6:w1219:errorcluster)  [unwired: 2 in, 1 out]
                        }
                        frame #1 {
                          n677 = while {
                            tunnel: w1222 -> [w1223]
                            i -> [w1224]
                            stop <- w1226 continue-if-true
                            n678 = GPIB Serial Poll(0:w1223) -> (2:w1228:i16)  [unwired: 1 in, 2 out]
                            n679 = Less?(x=w1228, y=i16 128) -> (x < y?=w1226:bool)
                            n680 = Wait (ms)(milliseconds to wait=u32 50) -> ()  [unwired: 1 out]
                            "Numeric 4" <- w1224
                          }
                        }
                        frame #2 {
                          w1229 = i16 2 ("mode (0)")
                          n681 = GPIB Read(0:w1231, 1:200 ("byte count"), 2:i16 2 ("mode (0)"), 3:w1242) -> (5:w1235:string)  [unwired: 1 in, 2 out]
                          n682 = Match Pattern(string=w1235, regular expression="C=") -> (after substring=w1234:string)  [unwired: 1 in, 3 out]
                          n683 = Match Pattern(string=w1234, regular expression="PF L=") -> (after substring=w1232:string)  [unwired: 1 in, 3 out]
                          n684 = Search/Split String(string=w1234, search string/char (-)=" ", offset (0)=w1229) -> (substring before match=w1239:string)  [unwired: 2 out]
                          n685 = Search/Split String(string=w1232, search string/char (-)=" ", offset (0)=w1229) -> (substring before match=w1238:string)  [unwired: 2 out]
                          n686 = Fract/Exp String To Number(string=w1238) -> (number=w1236:dbl)  [unwired: 3 in, 1 out]
                          n687 = Fract/Exp String To Number(string=w1239) -> (number=w1237:dbl)  [unwired: 3 in, 1 out]
                        }
                      }
                      n688 = Build Array (concatenate)(w1217, w1215) -> (w1214:dbl[])
                      n689 = Build Array (concatenate)(w1214, w1212) -> (w1213:dbl[])
                    }
                  }
                  n690 = property on="array for data" class="Arr (strict)"("Value"=w1209) -> ()  [unwired: 2 in, 2 out]
                }
              }
              n691 = property on="Commute SorceMeter" class="RadioBtnsControl (strict)"() -> ("Value"=w857:enum32{"Radio Selection 1", "Radio Selection 2"})  [unwired: 2 in, 2 out]
              n692 = case shown="\"Radio Selection 1\", Default" w857 {
                tunnel: ["13" "14"] -> w860
                frame "Radio Selection 1", Default {
                }
                frame "Radio Selection 2" {
                }
              }
              n693 = GPIB Write(0:w860, 1:":READ?", 3:w859) -> (6:w861:errorcluster)  [unwired: 2 in, 1 out]
              n694 = GPIB Read(0:w860, 1:3200, 3:w861) -> (5:w864:string)  [unwired: 2 in, 2 out]
              n695 = String Subset(string=w864, length (rest)=13) -> (substring=w865:string)  [unwired: 1 in]
              n696 = Fract/Exp String To Number(string=w865) -> (number=w867:dbl)  [unwired: 3 in, 1 out]
              n697 = Multiply(x=w867, y=-1.0) -> (x*y=w872:dbl)
              n698 = Number To Fractional String(number=w872) -> (F-format string=w869:string)  [unwired: 3 in]
              n699 = Concatenate Strings(":INIT:IMM; :SOUR:VOLT:LEV:IMM:AMPL " ("data"), w869) -> (w870:string)
              n700 = GPIB Write(0:w860, 1:w870) -> (6:w858:errorcluster)  [unwired: 3 in, 1 out]
            }
          }
        }
        frame False {
          # "all measurements are done in this stacked sequence; reading from each device is recorded to \"array for data\""
          n701 = stacked-sequence {
            tunnel: w1245 -> [w1247 _ _ _ _ _ _ _ _ _ _ _ _ _ _ _ _ _ _ _ _ _ _ _ _ _]
            tunnel: [w1247 _ _ _ _ _ _ _ _ _ _ _ _ _ _ _ _ _ _ _ _ _ _ _ _ _] -> w1246
            frame #0 {
              # "check if oscillator on \nlock-in (address 1)\nis to be measured"
              n702 = property on="Current is:" class="RadioBtnsControl (strict)"() -> ("Value"=w1250:T1)  [unwired: 2 in, 2 out]
              n703 = property on="array for data" class="Arr (strict)"() -> ("Value"=w1249:dbl[])  [unwired: 2 in, 2 out]
              n704 = Equal?(x=w1250, y=1) -> (x = y?=w1251:bool)
              n705 = case shown="True" w1251 {
                tunnel: w1249 -> [w1253 w1261]
                tunnel: [w1253 w1260] -> w1248
                frame False {
                  # "we are not measuring oscillator from\nlock-in (address 1)"
                }
                frame True {
                  w1257 = "1"
                  # "we are  measuring oscillator"
                  n706 = GPIB Write(0:w1257, 1:"SLVL?") -> (6:w1258:errorcluster)  [unwired: 3 in, 1 out]
                  n707 = GPIB Read(0:w1257, 1:3200, 3:w1258) -> (5:w1255:string)  [unwired: 2 in, 2 out]
                  n708 = Fract/Exp String To Number(string=w1255) -> (number=w1254:dbl)  [unwired: 3 in, 1 out]
                  n709 = Build Array (concatenate)(w1261, w1254) -> (w1260:dbl[])
                }
              }
              n710 = property on="array for data" class="Arr (strict)"("Value"=w1248) -> ()  [unwired: 2 in, 2 out]
            }
            frame #1 {
              # "check if in-phase\nsignal on lock-in \n(address 1) is to\nbe measured"
              n711 = property on="array for data" class="Arr (strict)"() -> ("Value"=w1264:dbl[])  [unwired: 2 in, 2 out]
              n712 = property on="Addr 1 lock-in" class="Bool (strict)"() -> ("Value"=w1262:bool)  [unwired: 2 in, 2 out]
              n713 = case shown="True" w1262 {
                tunnel: w1264 -> [w1265 w1273]
                tunnel: [w1265 w1272] -> w1263
                frame False {
                  # "we are not measuring in phase signal on lock-in (address 1)"
                }
                frame True {
                  w1270 = "1"
                  # "we are  measuring lock-in (address 1), in phase"
                  n714 = GPIB Write(0:w1270, 1:"OUTP?1") -> (6:w1271:errorcluster)  [unwired: 3 in, 1 out]
                  n715 = GPIB Read(0:w1270, 1:3200, 3:w1271) -> (5:w1268:string)  [unwired: 2 in, 2 out]
                  n716 = Fract/Exp String To Number(string=w1268) -> (number=w1267:dbl)  [unwired: 3 in, 1 out]
                  n717 = Build Array (concatenate)(w1273, w1267) -> (w1272:dbl[])
                }
              }
              n718 = property on="array for data" class="Arr (strict)"("Value"=w1263) -> ()  [unwired: 2 in, 2 out]
            }
            frame #2 {
              # "check if out-of-phase\nsignal on lock-in \n(address 1) is to\nbe measured"
              n719 = property on="Addr 1 lock-in oop" class="Bool (strict)"() -> ("Value"=w1274:bool)  [unwired: 2 in, 2 out]
              n720 = property on="array for data" class="Arr (strict)"() -> ("Value"=w1276:dbl[])  [unwired: 2 in, 2 out]
              n721 = case shown="False" w1274 {
                tunnel: w1276 -> [w1277 w1285]
                tunnel: [w1277 w1284] -> w1275
                frame False {
                  # "we are not measuring out-of-phase signal on lock-in (address 1)"
                }
                frame True {
                  w1282 = "1"
                  # "we are  measuring lock-in (address 1), out-of-phase signal"
                  n722 = GPIB Write(0:w1282, 1:"OUTP?2") -> (6:w1283:errorcluster)  [unwired: 3 in, 1 out]
                  n723 = GPIB Read(0:w1282, 1:3200, 3:w1283) -> (5:w1280:string)  [unwired: 2 in, 2 out]
                  n724 = Fract/Exp String To Number(string=w1280) -> (number=w1279:dbl)  [unwired: 3 in, 1 out]
                  n725 = Build Array (concatenate)(w1285, w1279) -> (w1284:dbl[])
                }
              }
              n726 = property on="array for data" class="Arr (strict)"("Value"=w1275) -> ()  [unwired: 2 in, 2 out]
            }
            frame #3 {
              # "check if in-phase\nsignal on lock-in \n(address 2) is to\nbe measured"
              n727 = property on="Addr 2 lock-in" class="Bool (strict)"() -> ("Value"=w1286:bool)  [unwired: 2 in, 2 out]
              n728 = property on="array for data" class="Arr (strict)"() -> ("Value"=w1288:dbl[])  [unwired: 2 in, 2 out]
              n729 = case shown="False" w1286 {
                tunnel: w1288 -> [w1289 w1297]
                tunnel: [w1289 w1296] -> w1287
                frame False {
                  # "we are not measuring in phase signal on lock-in (address 2)"
                }
                frame True {
                  w1294 = "2"
                  # "we are  measuring lock-in (address 2), in phase"
                  n730 = GPIB Write(0:w1294, 1:"OUTP?1") -> (6:w1295:errorcluster)  [unwired: 3 in, 1 out]
                  n731 = GPIB Read(0:w1294, 1:3200, 3:w1295) -> (5:w1292:string)  [unwired: 2 in, 2 out]
                  n732 = Fract/Exp String To Number(string=w1292) -> (number=w1291:dbl)  [unwired: 3 in, 1 out]
                  n733 = Build Array (concatenate)(w1297, w1291) -> (w1296:dbl[])
                }
              }
              n734 = property on="array for data" class="Arr (strict)"("Value"=w1287) -> ()  [unwired: 2 in, 2 out]
            }
            frame #4 {
              # "check if out-of-phase\nsignal on lock-in \n(address 2) is to\nbe measured"
              n735 = property on="Addr 2 lock-in oop" class="Bool (strict)"() -> ("Value"=w1298:bool)  [unwired: 2 in, 2 out]
              n736 = property on="array for data" class="Arr (strict)"() -> ("Value"=w1300:dbl[])  [unwired: 2 in, 2 out]
              n737 = case shown="False" w1298 {
                tunnel: w1300 -> [w1301 w1309]
                tunnel: [w1301 w1308] -> w1299
                tunnel: w1298 -> [_ _]
                frame False {
                  # "we are not measuring out-of-phase signal on lock-in (address 2)"
                }
                frame True {
                  w1306 = "2"
                  # "we are  measuring lock-in (address 2), out-of-phase"
                  n738 = GPIB Write(0:w1306, 1:"OUTP?2") -> (6:w1307:errorcluster)  [unwired: 3 in, 1 out]
                  n739 = GPIB Read(0:w1306, 1:3200, 3:w1307) -> (5:w1304:string)  [unwired: 2 in, 2 out]
                  n740 = Fract/Exp String To Number(string=w1304) -> (number=w1303:dbl)  [unwired: 3 in, 1 out]
                  n741 = Build Array (concatenate)(w1309, w1303) -> (w1308:dbl[])
                }
              }
              n742 = property on="array for data" class="Arr (strict)"("Value"=w1299) -> ()  [unwired: 2 in, 2 out]
            }
            frame #5 {
              # "check if in-phase\nsignal on lock-in \n(address 3) is to\nbe measured"
              n743 = property on="Addr 3 lock-in" class="Bool (strict)"() -> ("Value"=w1310:bool)  [unwired: 2 in, 2 out]
              n744 = property on="array for data" class="Arr (strict)"() -> ("Value"=w1312:dbl[])  [unwired: 2 in, 2 out]
              n745 = case shown="False" w1310 {
                tunnel: w1312 -> [w1313 w1321]
                tunnel: [w1313 w1320] -> w1311
                frame False {
                  # "we are not measuring in phase signal on lock-in (address 3)"
                }
                frame True {
                  w1318 = "3"
                  # "we are  measuring lock-in (address 3), in phase"
                  n746 = GPIB Write(0:w1318, 1:"OUTP?1") -> (6:w1319:errorcluster)  [unwired: 3 in, 1 out]
                  n747 = GPIB Read(0:w1318, 1:3200, 3:w1319) -> (5:w1316:string)  [unwired: 2 in, 2 out]
                  n748 = Fract/Exp String To Number(string=w1316) -> (number=w1315:dbl)  [unwired: 3 in, 1 out]
                  n749 = Build Array (concatenate)(w1321, w1315) -> (w1320:dbl[])
                }
              }
              n750 = property on="array for data" class="Arr (strict)"("Value"=w1311) -> ()  [unwired: 2 in, 2 out]
            }
            frame #6 {
              # "check if out-of-phase\nsignal on lock-in \n(address 3) is to\nbe measured"
              n751 = property on="Addr 3 lock-in oop" class="Bool (strict)"() -> ("Value"=w1322:bool)  [unwired: 2 in, 2 out]
              n752 = property on="array for data" class="Arr (strict)"() -> ("Value"=w1324:dbl[])  [unwired: 2 in, 2 out]
              n753 = case shown="False" w1322 {
                tunnel: w1324 -> [w1325 w1333]
                tunnel: [w1325 w1332] -> w1323
                frame False {
                  # "we are not measuring out-of-phase signal on lock-in (address 3)"
                }
                frame True {
                  w1330 = "3"
                  # "we are  measuring lock-in (address 3), out-of-phase"
                  n754 = GPIB Write(0:w1330, 1:"OUTP?2") -> (6:w1331:errorcluster)  [unwired: 3 in, 1 out]
                  n755 = GPIB Read(0:w1330, 1:3200, 3:w1331) -> (5:w1328:string)  [unwired: 2 in, 2 out]
                  n756 = Fract/Exp String To Number(string=w1328) -> (number=w1327:dbl)  [unwired: 3 in, 1 out]
                  n757 = Build Array (concatenate)(w1333, w1327) -> (w1332:dbl[])
                }
              }
              n758 = property on="array for data" class="Arr (strict)"("Value"=w1323) -> ()  [unwired: 2 in, 2 out]
            }
            frame #7 {
              # "check if in-phase\nsignal on lock-in \n(address 4) is to\nbe measured"
              n759 = property on="Addr 4 lock-in" class="Bool (strict)"() -> ("Value"=w1334:bool)  [unwired: 2 in, 2 out]
              n760 = property on="array for data" class="Arr (strict)"() -> ("Value"=w1336:dbl[])  [unwired: 2 in, 2 out]
              n761 = case shown="False" w1334 {
                tunnel: w1336 -> [w1337 w1345]
                tunnel: [w1337 w1344] -> w1335
                frame False {
                  # "we are not measuring in phase signal on lock-in (address 4)"
                }
                frame True {
                  w1342 = "4"
                  # "we are  measuring lock-in (address 4), in phase"
                  n762 = GPIB Write(0:w1342, 1:"OUTP?1") -> (6:w1343:errorcluster)  [unwired: 3 in, 1 out]
                  n763 = GPIB Read(0:w1342, 1:3200, 3:w1343) -> (5:w1340:string)  [unwired: 2 in, 2 out]
                  n764 = Fract/Exp String To Number(string=w1340) -> (number=w1339:dbl)  [unwired: 3 in, 1 out]
                  n765 = Build Array (concatenate)(w1345, w1339) -> (w1344:dbl[])
                }
              }
              n766 = property on="array for data" class="Arr (strict)"("Value"=w1335) -> ()  [unwired: 2 in, 2 out]
            }
            frame #8 {
              # "check if out-of-phase\nsignal on lock-in \n(address 4) is to\nbe measured"
              n767 = property on="Addr 4 lock-in oop" class="Bool (strict)"() -> ("Value"=w1346:bool)  [unwired: 2 in, 2 out]
              n768 = property on="array for data" class="Arr (strict)"() -> ("Value"=w1348:dbl[])  [unwired: 2 in, 2 out]
              n769 = case shown="False" w1346 {
                tunnel: w1348 -> [w1349 w1357]
                tunnel: [w1349 w1356] -> w1347
                frame False {
                  # "we are not measuring out-of-phase signal on lock-in (address 4)"
                }
                frame True {
                  w1354 = "4"
                  # "we are  measuring lock-in (address 4), out-of-phase"
                  n770 = GPIB Write(0:w1354, 1:"OUTP?2") -> (6:w1355:errorcluster)  [unwired: 3 in, 1 out]
                  n771 = GPIB Read(0:w1354, 1:3200, 3:w1355) -> (5:w1352:string)  [unwired: 2 in, 2 out]
                  n772 = Fract/Exp String To Number(string=w1352) -> (number=w1351:dbl)  [unwired: 3 in, 1 out]
                  n773 = Build Array (concatenate)(w1357, w1351) -> (w1356:dbl[])
                }
              }
              n774 = property on="array for data" class="Arr (strict)"("Value"=w1347) -> ()  [unwired: 2 in, 2 out]
            }
            frame #9 {
              # "check if in-phase\nsignal on lock-in \n(address 5) is to\nbe measured"
              n775 = property on="Addr 5 lock-in" class="Bool (strict)"() -> ("Value"=w1358:bool)  [unwired: 2 in, 2 out]
              n776 = property on="array for data" class="Arr (strict)"() -> ("Value"=w1360:dbl[])  [unwired: 2 in, 2 out]
              n777 = case shown="False" w1358 {
                tunnel: w1360 -> [w1361 w1369]
                tunnel: [w1361 w1368] -> w1359
                frame False {
                  # "we are not measuring in phase signal on lock-in (address 5)"
                }
                frame True {
                  w1366 = "5"
                  # "we are  measuring lock-in (address 5), in phase"
                  n778 = GPIB Write(0:w1366, 1:"OUTP?1") -> (6:w1367:errorcluster)  [unwired: 3 in, 1 out]
                  n779 = GPIB Read(0:w1366, 1:3200, 3:w1367) -> (5:w1364:string)  [unwired: 2 in, 2 out]
                  n780 = Fract/Exp String To Number(string=w1364) -> (number=w1363:dbl)  [unwired: 3 in, 1 out]
                  n781 = Build Array (concatenate)(w1369, w1363) -> (w1368:dbl[])
                }
              }
              n782 = property on="array for data" class="Arr (strict)"("Value"=w1359) -> ()  [unwired: 2 in, 2 out]
            }
            frame #10 {
              # "check if out-of-phase\nsignal on lock-in \n(address 5) is to\nbe measured"
              n783 = property on="Addr 5 lock-in oop" class="Bool (strict)"() -> ("Value"=w1370:bool)  [unwired: 2 in, 2 out]
              n784 = property on="array for data" class="Arr (strict)"() -> ("Value"=w1372:dbl[])  [unwired: 2 in, 2 out]
              n785 = case shown="False" w1370 {
                tunnel: w1372 -> [w1373 w1381]
                tunnel: [w1373 w1380] -> w1371
                frame False {
                  # "we are not measuring out-of-phase signal on lock-in (address 5)"
                }
                frame True {
                  w1378 = "5"
                  # "we are  measuring lock-in (address 5), out-of-phase"
                  n786 = GPIB Write(0:w1378, 1:"OUTP?2") -> (6:w1379:errorcluster)  [unwired: 3 in, 1 out]
                  n787 = GPIB Read(0:w1378, 1:3200, 3:w1379) -> (5:w1376:string)  [unwired: 2 in, 2 out]
                  n788 = Fract/Exp String To Number(string=w1376) -> (number=w1375:dbl)  [unwired: 3 in, 1 out]
                  n789 = Build Array (concatenate)(w1381, w1375) -> (w1380:dbl[])
                }
              }
              n790 = property on="array for data" class="Arr (strict)"("Value"=w1371) -> ()  [unwired: 2 in, 2 out]
            }
            frame #11 {
              # "check if voltage on \nChannel A of main\nKeithley 2614B \n(addr. 12) is to\nbe measured"
              n791 = property on="Voltage (Vk1)" class="Bool (strict)"() -> ("Value"=w1382:bool)  [unwired: 2 in, 2 out]
              n792 = property on="array for data" class="Arr (strict)"() -> ("Value"=w1384:dbl[])  [unwired: 2 in, 2 out]
              n793 = case shown="False" w1382 {
                tunnel: w1384 -> [w1385 w1393]
                tunnel: [w1385 w1392] -> w1383
                frame False {
                  # "we aren't measuring voltage \non main Keithley 2614B Channel A (addr. 12)"
                }
                frame True {
                  (unwired) 13
                  w1390 = "12"
                  # "we are measuring voltage of Channel A \non the main Keithley 2614B (addr. 12)"
                  n794 = GPIB Write(0:w1390, 1:"print(smua.measure.v())") -> (6:w1391:errorcluster)  [unwired: 3 in, 1 out]
                  n795 = GPIB Read(0:w1390, 1:3200, 3:w1391) -> (5:w1386:string)  [unwired: 2 in, 2 out]
                  n796 = Fract/Exp String To Number(string=w1386) -> (number=w1388:dbl)  [unwired: 3 in, 1 out]
                  n797 = Build Array (concatenate)(w1393, w1388) -> (w1392:dbl[])
                }
              }
              n798 = property on="array for data" class="Arr (strict)"("Value"=w1383) -> ()  [unwired: 2 in, 2 out]
            }
            frame #12 {
              # "check if current on \nChannel A of main\nKeithley 2614B \n(addr. 12) is to\nbe measured"
              n799 = property on="Current (Ik1)" class="Bool (strict)"() -> ("Value"=w1394:bool)  [unwired: 2 in, 2 out]
              n800 = property on="array for data" class="Arr (strict)"() -> ("Value"=w1396:dbl[])  [unwired: 2 in, 2 out]
              n801 = case shown="True" w1394 {
                tunnel: w1396 -> [w1397 w1399]
                tunnel: [w1397 w1398] -> w1395
                frame False {
                  # "we aren't measuring current \non main Keithley 2400 (addr. 12)"
                }
                frame True {
                  w1404 = "12"
                  # "we are measuring current of Channel A \non the main Keithley 2614B (addr. 12)"
                  n802 = GPIB Write(0:w1404, 1:"print(smua.measure.i())") -> (6:w1405:errorcluster)  [unwired: 3 in, 1 out]
                  n803 = GPIB Read(0:w1404, 1:3200, 3:w1405) -> (5:w1400:string)  [unwired: 2 in, 2 out]
                  n804 = Fract/Exp String To Number(string=w1400) -> (number=w1402:dbl)  [unwired: 3 in, 1 out]
                  n805 = Build Array (concatenate)(w1399, w1402) -> (w1398:dbl[])
                }
              }
              n806 = property on="array for data" class="Arr (strict)"("Value"=w1395) -> ()  [unwired: 2 in, 2 out]
            }
            frame #13 {
              # "check if voltage on \nChannel B of main\nKeithley 2614B \n(addr. 12) is to\nbe measured"
              n807 = property on="Voltage (Vk2)" class="Bool (strict)"() -> ("Value"=w1406:bool)  [unwired: 2 in, 2 out]
              n808 = property on="array for data" class="Arr (strict)"() -> ("Value"=w1408:dbl[])  [unwired: 2 in, 2 out]
              n809 = case shown="False" w1406 {
                tunnel: w1408 -> [w1409 w1411]
                tunnel: [w1409 w1410] -> w1407
                frame False {
                  # "we aren't measuring voltage \non additional Keithley 2400 (addr. 13)"
                }
                frame True {
                  w1416 = "12"
                  # "we are measuring voltage of Channel B \non the main Keithley 2614B (addr. 12)"
                  n810 = GPIB Write(0:w1416, 1:"print(smub.measure.v())") -> (6:w1417:errorcluster)  [unwired: 3 in, 1 out]
                  n811 = GPIB Read(0:w1416, 1:3200, 3:w1417) -> (5:w1412:string)  [unwired: 2 in, 2 out]
                  n812 = Fract/Exp String To Number(string=w1412) -> (number=w1414:dbl)  [unwired: 3 in, 1 out]
                  n813 = Build Array (concatenate)(w1411, w1414) -> (w1410:dbl[])
                }
              }
              n814 = property on="array for data" class="Arr (strict)"("Value"=w1407) -> ()  [unwired: 2 in, 2 out]
            }
            frame #14 {
              # "check if current on \nChannel B of main\nKeithley 2614B \n(addr. 12) is to\nbe measured"
              n815 = property on="Current (Ik2)" class="Bool (strict)"() -> ("Value"=w1418:bool)  [unwired: 2 in, 2 out]
              n816 = property on="array for data" class="Arr (strict)"() -> ("Value"=w1420:dbl[])  [unwired: 2 in, 2 out]
              n817 = case shown="False" w1418 {
                tunnel: w1420 -> [w1421 w1423]
                tunnel: [w1421 w1422] -> w1419
                frame False {
                  # "we aren't measuring current \non additional Keithley 2400 (addr. 13)"
                }
                frame True {
                  w1428 = "12"
                  # "we are measuring current of Channel B \non the main Keithley 2614B (addr. 12)"
                  n818 = GPIB Write(0:w1428, 1:"print(smub.measure.i())") -> (6:w1429:errorcluster)  [unwired: 3 in, 1 out]
                  n819 = GPIB Read(0:w1428, 1:3200, 3:w1429) -> (5:w1424:string)  [unwired: 2 in, 2 out]
                  n820 = Fract/Exp String To Number(string=w1424) -> (number=w1426:dbl)  [unwired: 3 in, 1 out]
                  n821 = Build Array (concatenate)(w1423, w1426) -> (w1422:dbl[])
                }
              }
              n822 = property on="array for data" class="Arr (strict)"("Value"=w1419) -> ()  [unwired: 2 in, 2 out]
            }
            frame #15 {
              # "check if voltage on \nadd. Keithley 2400 \n(addr. 14) is to\nbe measured"
              n823 = property on="Voltage (Vk3)" class="Bool (strict)"() -> ("Value"=w1430:bool)  [unwired: 2 in, 2 out]
              n824 = property on="array for data" class="Arr (strict)"() -> ("Value"=w1432:dbl[])  [unwired: 2 in, 2 out]
              n825 = case shown="False" w1430 {
                tunnel: w1432 -> [w1433 w1443]
                tunnel: [w1433 w1442] -> w1431
                frame False {
                  # "we aren't measuring voltage \non additional Keithley 2400 (addr. 14)"
                }
                frame True {
                  w1440 = "14"
                  # "we are measuring voltage \non additional Keithley 2400 (addr. 14)"
                  n826 = GPIB Write(0:w1440, 1:":READ?") -> (6:w1441:errorcluster)  [unwired: 3 in, 1 out]
                  n827 = GPIB Read(0:w1440, 1:3200, 3:w1441) -> (5:w1436:string)  [unwired: 2 in, 2 out]
                  n828 = String Subset(string=w1436, length (rest)=13) -> (substring=w1435:string)  [unwired: 1 in]
                  n829 = Fract/Exp String To Number(string=w1435) -> (number=w1438:dbl)  [unwired: 3 in, 1 out]
                  n830 = Build Array (concatenate)(w1443, w1438) -> (w1442:dbl[])
                }
              }
              n831 = property on="array for data" class="Arr (strict)"("Value"=w1431) -> ()  [unwired: 2 in, 2 out]
            }
            frame #16 {
              # "check if  current on \nadd. Keithley 2400 \n(addr. 14) is to\nbe measured"
              n832 = property on="Current (Ik3)" class="Bool (strict)"() -> ("Value"=w1444:bool)  [unwired: 2 in, 2 out]
              n833 = property on="array for data" class="Arr (strict)"() -> ("Value"=w1446:dbl[])  [unwired: 2 in, 2 out]
              n834 = case shown="False" w1444 {
                tunnel: w1446 -> [w1447 w1458]
                tunnel: [w1447 w1457] -> w1445
                frame False {
                  # "we aren't measuring current \non additional Keithley 2400 (addr. 14)"
                }
                frame True {
                  w1455 = "14"
                  # "we are measuring current\non additional Keithley 2400 (addr. 14)"
                  n835 = GPIB Write(0:w1455, 1:":READ?") -> (6:w1456:errorcluster)  [unwired: 3 in, 1 out]
                  n836 = GPIB Read(0:w1455, 1:3200, 3:w1456) -> (5:w1451:string)  [unwired: 2 in, 2 out]
                  n837 = String Subset(string=w1451, offset (0)=14, length (rest)=13) -> (substring=w1450:string)
                  n838 = Fract/Exp String To Number(string=w1450) -> (number=w1453:dbl)  [unwired: 3 in, 1 out]
                  n839 = Build Array (concatenate)(w1458, w1453) -> (w1457:dbl[])
                }
              }
              n840 = property on="array for data" class="Arr (strict)"("Value"=w1445) -> ()  [unwired: 2 in, 2 out]
            }
            frame #17 {
              # "check if 1st channel\non Keithley 2182 \n(addr. 15) is to\nbe measured"
              n841 = property on="Channel 1 (Vnano1)" class="Bool (strict)"() -> ("Value"=w1459:bool)  [unwired: 2 in, 2 out]
              n842 = property on="array for data" class="Arr (strict)"() -> ("Value"=w1461:dbl[])  [unwired: 2 in, 2 out]
              n843 = case shown="True" w1459 {
                tunnel: w1461 -> [w1462 w1470]
                tunnel: [w1462 w1469] -> w1460
                frame False {
                  # "we are not measuring 1st channel\non Keithley 2182 (addr. 15)"
                }
                frame True {
                  w1467 = "15"
                  # "we are measuring 1st channel\non Keithley 2182 (addr. 15)"
                  n844 = GPIB Write(0:w1467, 1:":SENSe:DATA:FRES?") -> (6:w1468:errorcluster)  [unwired: 3 in, 1 out]
                  n845 = GPIB Read(0:w1467, 1:200, 3:w1468) -> (5:w1463:string)  [unwired: 2 in, 2 out]
                  n846 = Fract/Exp String To Number(string=w1463) -> (number=w1465:dbl)  [unwired: 3 in, 1 out]
                  n847 = Build Array (concatenate)(w1470, w1465) -> (w1469:dbl[])
                }
              }
              n848 = property on="array for data" class="Arr (strict)"("Value"=w1460) -> ()  [unwired: 2 in, 2 out]
            }
            frame #18 {
              # "check if 2nd channel\non Keithley 2182 \n(addr. 15) is to\nbe measured"
              n849 = property on="Channel 2 (Vnano1b)" class="Bool (strict)"() -> ("Value"=w1471:bool)  [unwired: 2 in, 2 out]
              n850 = property on="array for data" class="Arr (strict)"() -> ("Value"=w1473:dbl[])  [unwired: 2 in, 2 out]
              n851 = case shown="False" w1471 {
                tunnel: w1473 -> [w1474 w1486]
                tunnel: [w1474 w1485] -> w1472
                frame False {
                  # "we are not measuring 1st channel\non Keithley 2182 (addr. 15)"
                }
                frame True {
                  w1477 = "15"
                  # "switching to channel 2 and then\nback to channel 1"
                  # "we are measuring 2nd channel\non Keithley 2182 (addr. 15)"
                  n852 = GPIB Write(0:w1477, 1:":SENSe:CHAN 2") -> (6:w1478:errorcluster)  [unwired: 3 in, 1 out]
                  n853 = GPIB Write(0:w1477, 1:":SENSe:DATA:FRES?", 3:w1478) -> (6:w1484:errorcluster)  [unwired: 2 in, 1 out]
                  n854 = GPIB Read(0:w1477, 1:200, 3:w1484) -> (5:w1480:string, 7:w1476:errorcluster)  [unwired: 2 in, 1 out]
                  n855 = GPIB Write(0:w1477, 1:":SENSe:CHAN 1", 3:w1476) -> ()  [unwired: 2 in, 2 out]
                  n856 = Fract/Exp String To Number(string=w1480) -> (number=w1482:dbl)  [unwired: 3 in, 1 out]
                  n857 = Build Array (concatenate)(w1486, w1482) -> (w1485:dbl[])
                }
              }
              n858 = property on="array for data" class="Arr (strict)"("Value"=w1472) -> ()  [unwired: 2 in, 2 out]
            }
            frame #19 {
              # "check if 1st channel\non Keithley 2182 \n(addr. 16) is to\nbe measured"
              n859 = property on="Channel 1 (Vnano2)" class="Bool (strict)"() -> ("Value"=w1487:bool)  [unwired: 2 in, 2 out]
              n860 = property on="array for data" class="Arr (strict)"() -> ("Value"=w1489:dbl[])  [unwired: 2 in, 2 out]
              n861 = case shown="True" w1487 {
                tunnel: w1489 -> [w1490 w1498]
                tunnel: [w1490 w1497] -> w1488
                frame False {
                  # "we are not measuring 1st channel\non Keithley 2182 (addr. 16)"
                }
                frame True {
                  w1495 = "16"
                  # "we are measuring 1st channel\non Keithley 2182 (addr. 16)"
                  n862 = GPIB Write(0:w1495, 1:":SENSe:DATA:FRES?") -> (6:w1496:errorcluster)  [unwired: 3 in, 1 out]
                  n863 = GPIB Read(0:w1495, 1:200, 3:w1496) -> (5:w1491:string)  [unwired: 2 in, 2 out]
                  n864 = Fract/Exp String To Number(string=w1491) -> (number=w1493:dbl)  [unwired: 3 in, 1 out]
                  n865 = Build Array (concatenate)(w1498, w1493) -> (w1497:dbl[])
                }
              }
              n866 = property on="array for data" class="Arr (strict)"("Value"=w1488) -> ()  [unwired: 2 in, 2 out]
            }
            frame #20 {
              # "check if 2nd channel\non Keithley 2182 \n(addr. 16) is to\nbe measured"
              n867 = property on="Channel 2 (Vnano2b)" class="Bool (strict)"() -> ("Value"=w1499:bool)  [unwired: 2 in, 2 out]
              n868 = property on="array for data" class="Arr (strict)"() -> ("Value"=w1501:dbl[])  [unwired: 2 in, 2 out]
              n869 = case shown="False" w1499 {
                tunnel: w1501 -> [w1502 w1514]
                tunnel: [w1502 w1513] -> w1500
                frame False {
                  # "we are not measuring 1st channel\non Keithley 2182 (addr. 16)"
                }
                frame True {
                  w1505 = "16"
                  # "switching to channel 2 and then\nback to channel 1"
                  # "we are measuring 2nd channel\non Keithley 2182 (addr. 16)"
                  n870 = GPIB Write(0:w1505, 1:":SENSe:CHAN 2") -> (6:w1506:errorcluster)  [unwired: 3 in, 1 out]
                  n871 = GPIB Write(0:w1505, 1:":SENSe:DATA:FRES?", 3:w1506) -> (6:w1512:errorcluster)  [unwired: 2 in, 1 out]
                  n872 = GPIB Read(0:w1505, 1:200, 3:w1512) -> (5:w1508:string, 7:w1504:errorcluster)  [unwired: 2 in, 1 out]
                  n873 = GPIB Write(0:w1505, 1:":SENSe:CHAN 1", 3:w1504) -> ()  [unwired: 2 in, 2 out]
                  n874 = Fract/Exp String To Number(string=w1508) -> (number=w1510:dbl)  [unwired: 3 in, 1 out]
                  n875 = Build Array (concatenate)(w1514, w1510) -> (w1513:dbl[])
                }
              }
              n876 = property on="array for data" class="Arr (strict)"("Value"=w1500) -> ()  [unwired: 2 in, 2 out]
            }
            frame #21 {
              # "check if 1st channel\non Keithley 2182 \n(addr. 17) is to\nbe measured"
              n877 = property on="Channel 1 (Vnano3)" class="Bool (strict)"() -> ("Value"=w1515:bool)  [unwired: 2 in, 2 out]
              n878 = property on="array for data" class="Arr (strict)"() -> ("Value"=w1517:dbl[])  [unwired: 2 in, 2 out]
              n879 = case shown="False" w1515 {
                tunnel: w1517 -> [w1518 w1526]
                tunnel: [w1518 w1525] -> w1516
                frame False {
                  # "we are not measuring 1st channel\non Keithley 2182 (addr. 17)"
                }
                frame True {
                  w1523 = "17"
                  # "we are measuring 1st channel\non Keithley 2182 (addr. 17)"
                  n880 = GPIB Write(0:w1523, 1:":SENSe:DATA:FRES?") -> (6:w1524:errorcluster)  [unwired: 3 in, 1 out]
                  n881 = GPIB Read(0:w1523, 1:200, 3:w1524) -> (5:w1519:string)  [unwired: 2 in, 2 out]
                  n882 = Fract/Exp String To Number(string=w1519) -> (number=w1521:dbl)  [unwired: 3 in, 1 out]
                  n883 = Build Array (concatenate)(w1526, w1521) -> (w1525:dbl[])
                }
              }
              n884 = property on="array for data" class="Arr (strict)"("Value"=w1516) -> ()  [unwired: 2 in, 2 out]
            }
            frame #22 {
              # "check if 2nd channel\non Keithley 2182 \n(addr. 17) is to\nbe measured"
              n885 = property on="Channel 2 (Vnano3b)" class="Bool (strict)"() -> ("Value"=w1527:bool)  [unwired: 2 in, 2 out]
              n886 = property on="array for data" class="Arr (strict)"() -> ("Value"=w1529:dbl[])  [unwired: 2 in, 2 out]
              n887 = case shown="False" w1527 {
                tunnel: w1529 -> [w1530 w1542]
                tunnel: [w1530 w1541] -> w1528
                frame False {
                  # "we are not measuring 1st channel\non Keithley 2182 (addr. 17)"
                }
                frame True {
                  w1533 = "17"
                  # "switching to channel 2 and then\nback to channel 1"
                  # "we are measuring 2nd channel\non Keithley 2182 (addr. 17)"
                  n888 = GPIB Write(0:w1533, 1:":SENSe:CHAN 2") -> (6:w1534:errorcluster)  [unwired: 3 in, 1 out]
                  n889 = GPIB Write(0:w1533, 1:":SENSe:DATA:FRES?", 3:w1534) -> (6:w1540:errorcluster)  [unwired: 2 in, 1 out]
                  n890 = GPIB Read(0:w1533, 1:200, 3:w1540) -> (5:w1536:string, 7:w1532:errorcluster)  [unwired: 2 in, 1 out]
                  n891 = GPIB Write(0:w1533, 1:":SENSe:CHAN 1", 3:w1532) -> ()  [unwired: 2 in, 2 out]
                  n892 = Fract/Exp String To Number(string=w1536) -> (number=w1538:dbl)  [unwired: 3 in, 1 out]
                  n893 = Build Array (concatenate)(w1542, w1538) -> (w1541:dbl[])
                }
              }
              n894 = property on="array for data" class="Arr (strict)"("Value"=w1528) -> ()  [unwired: 2 in, 2 out]
            }
            frame #23 {
              # "check if 1st \nthermometer on \nOxford ITC \n(address 24) \nis measured"
              n895 = property on="Thermometer 1 (T1)" class="Bool (strict)"() -> ("Value"=w1543:bool)  [unwired: 2 in, 2 out]
              n896 = property on="array for data" class="Arr (strict)"() -> ("Value"=w1545:dbl[])  [unwired: 2 in, 2 out]
              n897 = case shown="True" w1543 {
                tunnel: w1545 -> [w1546 w1558]
                tunnel: [w1546 w1557] -> w1544
                frame False {
                  # "we are not measuring temperature on\nthermometer 1 (addr. 24)"
                }
                frame True {
                  (unwired) "\r"
                  w1551 = refnum<visa-resource-name> "TCPIP0::192.168.128.2::7020::SOCKET" ("VISA resource name")
                  # "we are measuring temperature,\nthermometer 1 (addr. 24)"
                  n898 = Concatenate Strings("READ:DEV:MB1.T1:TEMP:SIG:TEMP" ("string"), "\n") -> (w1550:string)
                  n899 = VISA Write(VISA resource name=w1551, write buffer=w1550) -> (error out=w1556:errorcluster)  [unwired: 1 in, 2 out]
                  n900 = String Length(string=w1550) -> (length=w1547:i32)
                  n901 = VISA Read(VISA resource name=w1551, byte count=1024, error in (no error)=w1556) -> (read buffer=w1554:string)  [unwired: 3 out]
                  n902 = String Subset(string=w1554, offset (0)=w1547) -> (substring=w1553:string)  [unwired: 1 in]
                  n903 = Fract/Exp String To Number(string=w1553) -> (number=w1549:dbl)  [unwired: 3 in, 1 out]
                  n904 = Build Array (concatenate)(w1558, w1549) -> (w1557:dbl[])
                }
              }
              n905 = property on="array for data" class="Arr (strict)"("Value"=w1544) -> ()  [unwired: 2 in, 2 out]
            }
            frame #24 {
              # "check if 1st \nthermometer on \nOxford ITC \n(address 24) \nis measured"
              n906 = property on="Magnetic Field (B)" class="Bool (strict)"() -> ("Value"=w1559:bool)  [unwired: 2 in, 2 out]
              n907 = property on="array for data" class="Arr (strict)"() -> ("Value"=w1561:dbl[])  [unwired: 2 in, 2 out]
              n908 = case shown="True" w1559 {
                tunnel: w1561 -> [w1562 w1574]
                tunnel: [w1562 w1573] -> w1560
                frame False {
                  # "we are not measuringmagnetic field (addr. 25)"
                }
                frame True {
                  (unwired) "\r"
                  w1567 = refnum<visa-resource-name> "TCPIP0::192.168.128.3::7020::SOCKET" ("VISA resource name")
                  # "we are measuring magnetic field  (addr. 25)"
                  n909 = Concatenate Strings("READ:DEV:GRPZ:PSU:SIG:FLD" ("string"), "\n") -> (w1566:string)
                  n910 = VISA Write(VISA resource name=w1567, write buffer=w1566) -> (error out=w1572:errorcluster)  [unwired: 1 in, 2 out]
                  n911 = String Length(string=w1566) -> (length=w1563:i32)
                  n912 = VISA Read(VISA resource name=w1567, byte count=1024, error in (no error)=w1572) -> (read buffer=w1570:string)  [unwired: 3 out]
                  n913 = String Subset(string=w1570, offset (0)=w1563) -> (substring=w1569:string)  [unwired: 1 in]
                  n914 = Fract/Exp String To Number(string=w1569) -> (number=w1565:dbl)  [unwired: 3 in, 1 out]
                  n915 = Build Array (concatenate)(w1574, w1565) -> (w1573:dbl[])
                }
              }
              n916 = property on="array for data" class="Arr (strict)"("Value"=w1560) -> ()  [unwired: 2 in, 2 out]
            }
            frame #25 {
              # "check if capacitance\nand loss (address 28)\nare measured"
              n917 = property on="Capacitance (C) and Loss (L)" class="Bool (strict)"() -> ("Value"=w1575:bool)  [unwired: 2 in, 2 out]
              n918 = property on="array for data" class="Arr (strict)"() -> ("Value"=w1577:dbl[])  [unwired: 2 in, 2 out]
              n919 = case shown="False" w1575 {
                tunnel: w1577 -> [w1578 w1584]
                tunnel: [w1578 w1580] -> w1576
                frame False {
                  # "we are not measuringmagnetic capacitance (addr. 28)"
                }
                frame True {
                  # "we are measuring capacitance and loss  (addr. 28)"
                  n920 = stacked-sequence {
                    seq-local: [w1586 _ _] -> [_ _ w1609]
                    tunnel: [_ _ w1603] -> w1579
                    tunnel: [_ _ w1604] -> w1582
                    tunnel: "28" ("data") -> [w1585 w1589 w1598]
                    frame #0 {
                      n921 = GPIB Write(0:w1585, 1:"SINGLE" ("data"), 2:i16 0 ("mode (0)")) -> (6:w1586:errorcluster)  [unwired: 2 in, 1 out]
                    }
                    frame #1 {
                      n922 = while {
                        tunnel: w1589 -> [w1590]
                        i -> [w1591]
                        stop <- w1593 continue-if-true
                        n923 = GPIB Serial Poll(0:w1590) -> (2:w1595:i16)  [unwired: 1 in, 2 out]
                        n924 = Less?(x=w1595, y=i16 128) -> (x < y?=w1593:bool)
                        n925 = Wait (ms)(milliseconds to wait=u32 50) -> ()  [unwired: 1 out]
                        "Numeric 3" <- w1591
                      }
                    }
                    frame #2 {
                      w1596 = i16 2 ("mode (0)")
                      n926 = GPIB Read(0:w1598, 1:200 ("byte count"), 2:i16 2 ("mode (0)"), 3:w1609) -> (5:w1602:string)  [unwired: 1 in, 2 out]
                      n927 = Match Pattern(string=w1602, regular expression="C=") -> (after substring=w1601:string)  [unwired: 1 in, 3 out]
                      n928 = Match Pattern(string=w1601, regular expression="PF L=") -> (after substring=w1599:string)  [unwired: 1 in, 3 out]
                      n929 = Search/Split String(string=w1601, search string/char (-)=" ", offset (0)=w1596) -> (substring before match=w1606:string)  [unwired: 2 out]
                      n930 = Search/Split String(string=w1599, search string/char (-)=" ", offset (0)=w1596) -> (substring before match=w1605:string)  [unwired: 2 out]
                      n931 = Fract/Exp String To Number(string=w1605) -> (number=w1603:dbl)  [unwired: 3 in, 1 out]
                      n932 = Fract/Exp String To Number(string=w1606) -> (number=w1604:dbl)  [unwired: 3 in, 1 out]
                    }
                  }
                  n933 = Build Array (concatenate)(w1584, w1582) -> (w1581:dbl[])
                  n934 = Build Array (concatenate)(w1581, w1579) -> (w1580:dbl[])
                }
              }
              n935 = property on="array for data" class="Arr (strict)"("Value"=w1576) -> ()  [unwired: 2 in, 2 out]
            }
          }
        }
      }
      n936 = property on="array for data" class="Arr (strict)"(error in=w440) -> ("Value"=w418:dbl[])  [unwired: 1 in, 2 out]
      n937 = while {
        shift-right: [w1623] -> w414
        shift-left: w418 -> [w1625]
        i -> [w1624]
        stop <- w1628 stop-if-true
        # "loop goes through the list of all measured parameters\nif some columns are identified as current or resistance\nthey are recalculated according to selected or entered parameters"
        n938 = Increment(x=w1624) -> (x+1=w1629:i32)
        n939 = property on="Ring" class="Ring (strict)"() -> ("Strings []"=w1627:string[])  [unwired: 2 in, 2 out]
        n940 = Index Array(array=w1627, index=w1624) -> (element=w1626:string)
        n941 = property on="Ring" class="Ring (strict)"() -> ("NumItems"=w1630:u32)  [unwired: 2 in, 2 out]
        n942 = case shown="\"False\", Default" w1626 {
          tunnel: w1625 -> [w1636 w1646 w1656 w1663]
          tunnel: w1624 -> [w1634 w1643 w1654 _]
          tunnel: [w1635 w1644 w1655 w1663] -> w1623
          frame "I" {
            n943 = property on="Current is:" class="RadioBtnsControl (strict)"() -> ("Value"=w1632:T1)  [unwired: 2 in, 2 out]
            n944 = case shown="\"Radio Selection 2\"" w1632 {
              tunnel: ["Ring 3" "Ring 2"] -> w1631
              frame "Radio Selection 3", Default {
              }
              frame "Radio Selection 2" {
              }
            }
            n945 = Index Array(array=w1636, index=w1634) -> (element=w1637:dbl)
            n946 = Power Of 10(x=w1631) -> (10^x=w1640:dbl)
            n947 = Multiply(x=1000.0, y=w1640) -> (x*y=w1638:dbl)
            n948 = Divide(x=w1637, y=w1638) -> (x/y=w1633:dbl)
            "Numeric Current" <- w1633
            n949 = Replace Array Subset(array=w1636, new element=w1633, index=w1634) -> (w1635:dbl[])
          }
          frame "Ioop" {
            n950 = property on="Ring 3" class="Ring (strict)"() -> ("Value"=w1645:u16)  [unwired: 2 in, 2 out]
            n951 = Index Array(array=w1646, index=w1643) -> (element=w1648:dbl)
            n952 = Power Of 10(x=w1645) -> (10^x=w1651:dbl)
            n953 = Multiply(x=1000.0, y=w1651) -> (x*y=w1649:dbl)
            n954 = Divide(x=w1648, y=w1649) -> (x/y=w1647:dbl)
            n955 = Replace Array Subset(array=w1646, new element=w1647, index=w1643) -> (w1644:dbl[])
          }
          frame "R1", "R1oop", "R2", "R2oop", "R3", "R3oop", "R4", "R4oop", "R5", "R5oop" {
            n956 = property on="Current is:" class="RadioBtnsControl (strict)"() -> ("Value"=w1653:T1)  [unwired: 2 in, 2 out]
            n957 = case shown="\"Radio Selection 2\", Default" w1653 {
              tunnel: [w1659 w1662] -> w1652
              frame "Radio Selection 1" {
                n958 = Divide(x="Fixed Current mkA", y=1000000.0) -> (x/y=w1659:dbl)
              }
              frame "Radio Selection 2", Default {
                n959 = property on="Numeric Current" class="DigNum (strict)"() -> ("Value"=w1662:dbl)  [unwired: 2 in, 2 out]
              }
            }
            n960 = Index Array(array=w1656, index=w1654) -> (element=w1658:dbl)
            n961 = Divide(x=w1658, y=w1652) -> (x/y=w1657:dbl)
            n962 = Replace Array Subset(array=w1656, new element=w1657, index=w1654) -> (w1655:dbl[])
          }
          frame "False", Default {
          }
        }
        n963 = Less?(x=w1630, y=w1629) -> (x < y?=w1628:bool)
      }
      n964 = Subtract(x="Target Voltage, V", y=w424) -> (x-y=w427:dbl)
      n965 = Divide(x="Sweep rate, V/min", y=60.0) -> (x/y=w436:dbl)
      n966 = Multiply(x=w436, y="Time btw \npoints, sec") -> (x*y=w419:dbl)
      n967 = Sign(1:w427) -> (0:w420:dbl)
      n968 = Multiply(x=w420, y=w419) -> (x*y=w412:dbl)
      n969 = property on="points at each Vg" class="DigNum (strict)"() -> ("Value"=w411:i32)  [unwired: 2 in, 2 out]
      n970 = To Double Precision Float(number=w411) -> (double precision float=w410:dbl)
      n971 = Multiply(x=w410, y=w412) -> (x*y=w409:dbl)
      n972 = property on="Commutator" class="Bool (strict)"() -> ("Value"=w403:bool)  [unwired: 2 in, 2 out]
      n973 = property on="Data file:" class="Path"() -> ("Value"=w416:path)  [unwired: 2 in, 2 out]
      n974 = Divide(x=w427, y=w409) -> (x/y=w434:dbl)
      n975 = case shown="False" w403 {
        tunnel: w421 -> [w454 w465]
        tunnel: w405 -> [w449 w459]
        tunnel: [w441 w458] -> w402
        frame True {
          # "calculate deliberate time delay for the next step"
          n976 = Subtract(x=w454, y=w449) -> (x-y=w447:u32)
          n977 = property on="Delib Time delay" class="DigNum (strict)"() -> ("Value"=w448:i32)  [unwired: 2 in, 2 out]
          n978 = property on="Time btw \npoints, sec" class="DigNum (strict)"() -> ("Value"=w453:dbl)  [unwired: 2 in, 2 out]
          n979 = Subtract(x=w447, y=w448) -> (x-y=w446:u32)
          n980 = Multiply(x=w453, y=1000.0) -> (x*y=w451:dbl)
          n981 = To Long Integer(number=w451) -> (32bit integer=w450:i32)
          n982 = Greater?(x=w450, y=w446) -> (0:w443:bool)
          n983 = Subtract(x=w450, y=w446) -> (x-y=w445:u32)
          n984 = Divide(x=w445, y=2) -> (x/y=w442:dbl)
          n985 = case shown="False" w443 {
            tunnel: w442 -> [_ w457]
            tunnel: [0 w456] -> w441
            frame False {
            }
            frame True {
              n986 = To Long Integer(number=w457) -> (32bit integer=w456:i32)
            }
          }
        }
        frame False {
          # "calculate deliberate time delay for the next step"
          n987 = Subtract(x=w465, y=w459) -> (x-y=w462:u32)
          n988 = property on="Time btw \npoints, sec" class="DigNum (strict)"() -> ("Value"=w464:dbl)  [unwired: 2 in, 2 out]
          n989 = Multiply(x=w464, y=1000.0) -> (x*y=w461:dbl)
          n990 = To Long Integer(number=w461) -> (32bit integer=w460:i32)
          n991 = Greater?(x=w460, y=w462) -> ()  [unwired: 1 out]
          n992 = Subtract(x=w460, y=w462) -> (x-y=w458:u32)
        }
      }
      "Delib Time delay" <- w402
      n993 = Decrement(x=w434) -> (x-1=w433:dbl)
      n994 = Absolute Value(x=w427) -> (abs(x)=w429:dbl)
      n995 = Build Array (concatenate)(w439, w414) -> (w413:dbl[][])
      n996 = Greater Than 0?(x=w433) -> (x > 0?=w432:bool)
      n997 = property on="array for data" class="Arr (strict)"("Value"=w414) -> ()  [unwired: 2 in, 2 out]
      n998 = call-poly <vilib>:"Write To Spreadsheet File.vi"("format (%.3f)"="%#g", "append to file? (new file:F)"=TRUE, "1D data"=w414, "file path (dialog if empty)"=w416) -> ()  [unwired: 4 in, 1 out]
      n999 = Less?(x=w429, y=1e-06) -> (x < y?=w426:bool)
      n1000 = flat-sequence {
        tunnel: [w1622] -> w421
        tunnel: w413 -> [w1616]
        frame #0 {
          # "time is mesured at the end of the cycle\nto adjust a delay time"
          # "this part plots selected measurements"
          n1001 = Tick Count (ms)() -> (millisecond timer value=w1622:u32)
          n1002 = Index Array(array=w1616, index (col)="Ring") -> (element=w1621:dbl[])  [unwired: 1 in]
          n1003 = Index Array(array=w1616, index (col)=0) -> (element=w1619:dbl[])  [unwired: 1 in]
          n1004 = Bundle(w1619, w1621) -> (→"XY Graph":cluster{dbl[], dbl[]})  [unwired: 1 in]
        }
      }
      n1005 = case shown="True" w432 {
        tunnel: w424 -> [_ w1667]
        tunnel: w409 -> [_ w1666]
        tunnel: [w1664 w1665] -> w431
        frame False {
          # "if next step is too long\nuse target voltage"
          n1006 = property on="Target Voltage, V" class="DigNum (strict)"() -> ("Value"=w1664:dbl)  [unwired: 2 in, 2 out]
        }
        frame True {
          # "add increment to\nthe current Vg"
          n1007 = Add(x=w1666, y=w1667) -> (x+y=w1665:dbl)
        }
      }
    }
    n1008 = Number To Fractional String(number=w381) -> (F-format string=w386:string)  [unwired: 3 in]
    n1009 = property on="Main Keithly2614B address" class="Str"() -> ("Value"=w384:string)  [unwired: 2 in, 2 out]
    n1010 = Concatenate Strings("smua.source.levelv = " ("data"), w386) -> (w385:string)
    n1011 = Equal?(x=w379, y="optional Bias (V)") -> (x = y?=w382:bool)
    n1012 = case shown="True" w382 {
      tunnel: "optional Bias (V)" -> [w393 _]
      tunnel: w381 -> [w394 _]
      frame False {
        n1013 = Multiply(x=w394, y=22.62) -> (x*y=w395:dbl)
        n1014 = Number To Fractional String(number=w393) -> (F-format string=w401:string)  [unwired: 3 in]
        n1015 = Add(x=w393, y=w395) -> ()  [unwired: 1 out]
        n1016 = Concatenate Strings(":INIT:IMM; :SOUR:VOLT:LEV:IMM:AMPL " ("data"), w401) -> (w400:string)
        n1017 = property on="optional Bias (V)" class="DigNum (strict)"("Visible"=TRUE) -> ()  [unwired: 2 in, 2 out]
        n1018 = GPIB Write(0:"13", 1:w400) -> ()  [unwired: 3 in, 2 out]
      }
      frame True {
      }
    }
    n1019 = GPIB Write(0:w384, 1:w385) -> ()  [unwired: 3 in, 2 out]
  }
  "Array 2" <- w16
  n1020 = Concatenate Strings(w6, w2, w1, w3, w2, w1) -> (w18:string)
  "String" <- w18
  n1021 = Write to Text File(file (use dialog)=w19, text=w18) -> ()  [unwired: 2 in, 3 out]
  n1022 = property on="optional Bias (V)" class="DigNum (strict)"("Value"=w14, "Visible"=FALSE) -> ()  [unwired: 2 in, 2 out]
